vi "Automated Pressure Control v20.vi"() -> ()   [LabVIEW 2011]
uses:
  <vilib>/LabVIEW Interface for Arduino/Type Defs/Pin Mode.ctl
  <vilib>/LabVIEW Interface for Arduino/Type Defs/Arduino Resource.ctl
  <vilib>/LabVIEW Interface for Arduino/Type Defs/Board Type.ctl
  orders/Firgelli motor/LAC_Software_V2/Firgelli Labview Example/Firgelli_LAC_LabVIEWsourceVer8_2/typeDefs/controlValues.ctl
  <vilib>/vision/Avi1.llb/AviRefnum.ctl
  <vilib>/LabVIEW Interface for Arduino/LabVIEW Interface for Arduino.lvlib
  <vilib>/vision/NI_Vision_Development_Module.lvlib
panel:
  out "Balancing":bool
  out "pArray":dbl[](array[numeric])
  in  "Transducer (psi)":dbl(ring)=1.0 items=["+/- .18 psi"=1.0, "+/- .36 psi"=2.0, "+/- 1.08 psi"=3.0]
  in  "Velocity (%)":dbl(slide)=50.0 min=0.0 max=100.0 step=0.01 scale=0.0..100.0 scale format="%02.2f"
  in  "Digital I/O Pin":u8=4
  in  "VentValveOpen?":bool
  out "selected path":path
  out "Capture Video? 2":bool
  out "VidStarted?":bool
  out "loopTimes":dbl[](array[numeric])
  out "Avi Refnum":T1
  in  "Capture Video?":bool
  out "loop exec time (ms)":u32
  out "frameSize":cluster{"Height":i32, "Width":i32}
  out "ROIYDim":dbl
  out "ROIXDim":dbl
  in  "Clear ROI":bool
  in  "Accept ROI":bool
  out "ROI":T2(plugin-control)
  out "error out":errorcluster caption="error"
  in  "Camera ID":u32
  in  "Stopp":bool
  out "FPS":dbl=6.258409738085552
  out "Width":i32=640
  out "Height":i32=480
  in  "Autogain":bool=TRUE
  in  "Master Gain":i32(slide) min=0 max=100 scale=0.0..100.0
  in  "Hotpixel correction":bool
  in  "Blacklevel compensation":bool
  in  "Edge Filter":i32(ring)=2 items=["High"=1, "Low"=2]
  in  "Edge Filter Enable / Disable":bool
  in  "Exposure time":dbl(slide)=33.21525 min=0.045771428571428574 max=49.06697142857143 step=0.045771428571428574 scale=0.045771428571428574..49.06697142857143 scale format="%#.3g"
  in  "Pixel clock":i32(slide)=20 min=5 max=43 scale=5.0..43.0
  in  "Frame rate":dbl(slide)=30.0 min=7.11187838119018 max=20.361314433379523 step=4.577142857142857e-05 scale=7.11187838119018..20.361314433379523 scale format="%^#_3g"
  in  "Blacklevel Offset":i32(slide) min=0 max=255 scale=0.0..255.0
  out "Bits/Pixel":i32=8
  in  "Syringe (mL)":dbl(ring)=2.0 items=[".5 mL"=2.0, "1 mL"=1.0, "3 mL"=3.0]
  out "LastPosition":dbl
  in  "Meas. Pressure":dbl=0.2
  in  "Accuracy (mm)":dbl(slide)=1.0 min=0.0 max=50.0 step=1e-06 scale=0.0..50.0 scale format="%.2f"
  in  "Position (mm) 2":dbl(slide)=40.0 min=0.0 max=50.0 step=0.1 scale=0.0..50.0 scale format="%.2f"
  in  "Position (mm)":dbl(slide)=35.0 min=0.0 max=50.0 step=0.3 scale=0.0..50.0 scale format="%.2f"
  in  "Balance":bool
  out "Pressure (psi)":dbl(graph) caption="Waveform Chart"
  out "Pressure (psi)":dbl
  out "Actuator Position (mm)":dbl(graph)
  in  "updateRate":i32=100 caption="Update Rate (mSec)"
  out "Control Values":T3
  in  "stop":bool
  out "ArduinoError":errorcluster
  out "ArduinoHandle":T4={"VISA resource"="", "Board Type"=enum."Uno", "Connection Type"=enum."USB / Serial", "Bytes Per Packet (15)"=15}
  in  "Valve I/O Pin":u8=2
  in  "Pin Mode":T6=enum."Output"
  in  "VISA resource":refnum<visa-resource-name>="COM6"
  in  "Zero":bool
  out "PressureOffset":dbl
  in  "ValveOpen?":bool
  out "FirgelliError":errorcluster
  out "READ_HANDLE":u32 format="%04x"
  out "WRITE_HANDLE":u32 format="%04x"
  out "DLLver":string caption="DLL Version"
  in  "StartMeasure":bool
  in  "Balance Pressure":dbl=-0.035 min=-1.0 max=0.0 step=0.001
  in  "Initialize":bool
  in  "length":dbl=50.0 caption="Actuator Length (mm)"
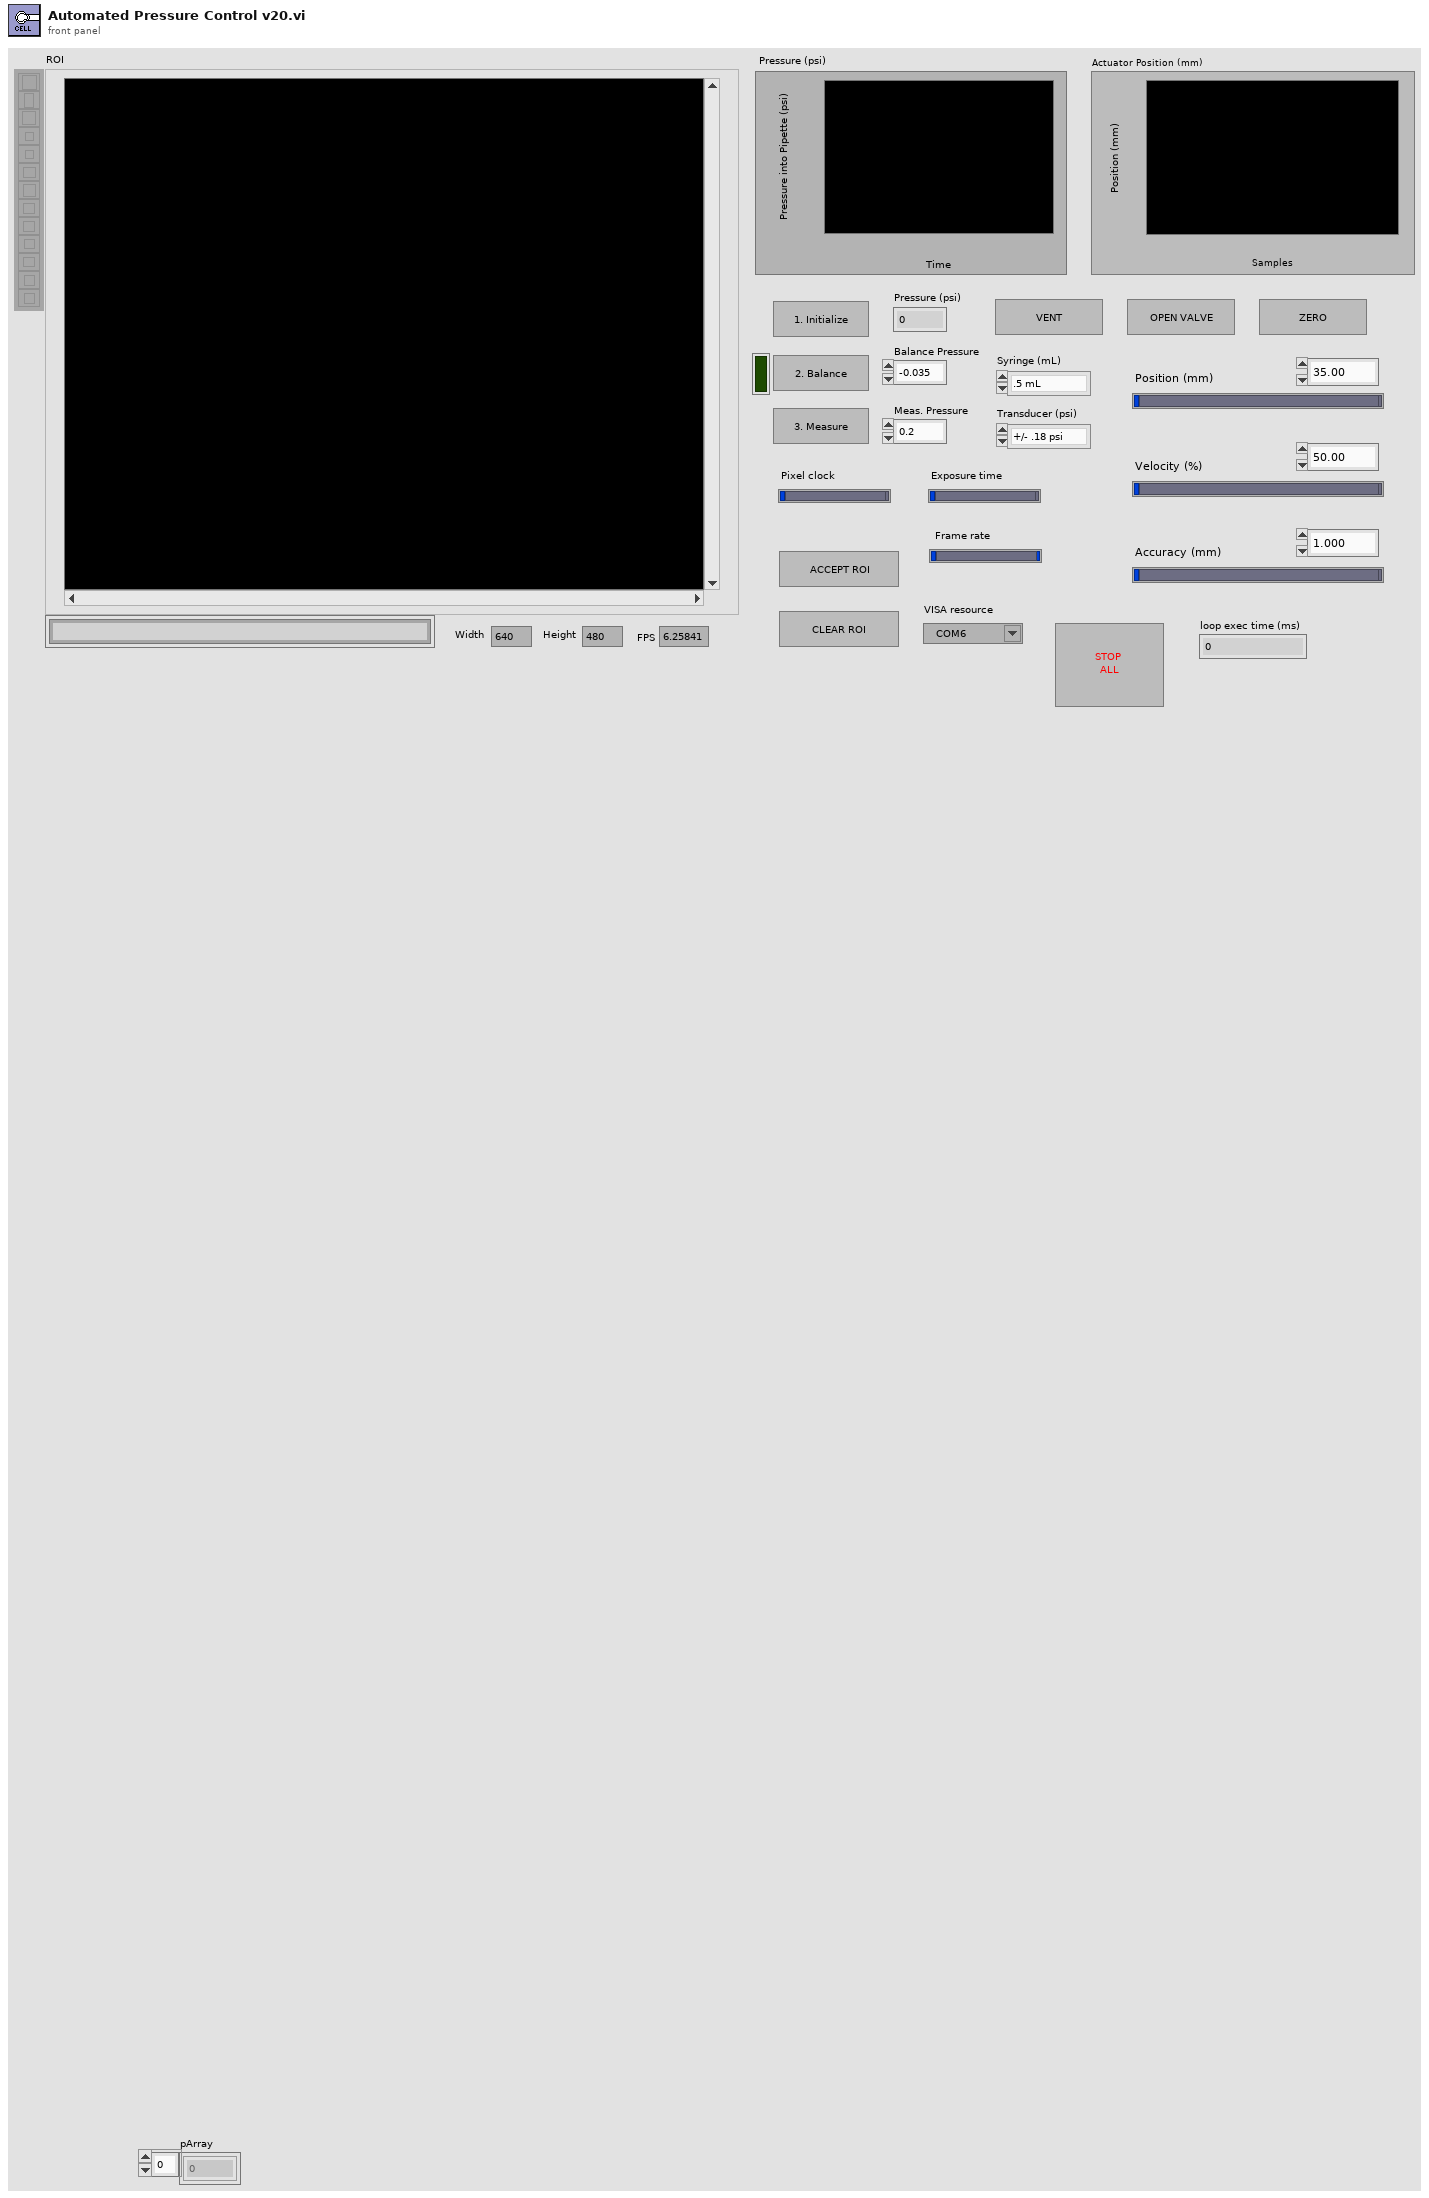
[diagram p1: front panel]
types:
  T1 = typedef "AviRefnum.ctl" = refnum<k1>
  T2 = typedef "IMAQ Image.ctl" = refnum<image>
  T3 = typedef "controlValues.ctl" = cluster{"Position":u16, "Velocity":u16, "Accuracy":u16, "Retract Limit":u16, "Extend Limit":u16}
  T4 = typedef "LabVIEW Interface for Arduino.lvlib/Arduino Resource.ctl" = cluster{"VISA resource":refnum<visa-resource-name>, "Board Type":T5, "Connection Type":enum8{"USB / Serial"}, "Bytes Per Packet (15)":u8}
  T5 = typedef "LabVIEW Interface for Arduino.lvlib/Board Type.ctl" = enum16{"Uno", "Dimuelanove w/Atmega 328", "Mega 2560"}
  T6 = typedef "LabVIEW Interface for Arduino.lvlib/Pin Mode.ctl" = enum8{"Input", "Output"}
  T7 = cluster{"Global Rectangle":i32[], "Contours":cluster{"Contour Type":u32, "ROI Type":u32, "Points":i32[]}[]}
  T8 = cluster{"x1Left":i32, "y1Top":i32, "x2Right":i32, "y2Bottom":i32}
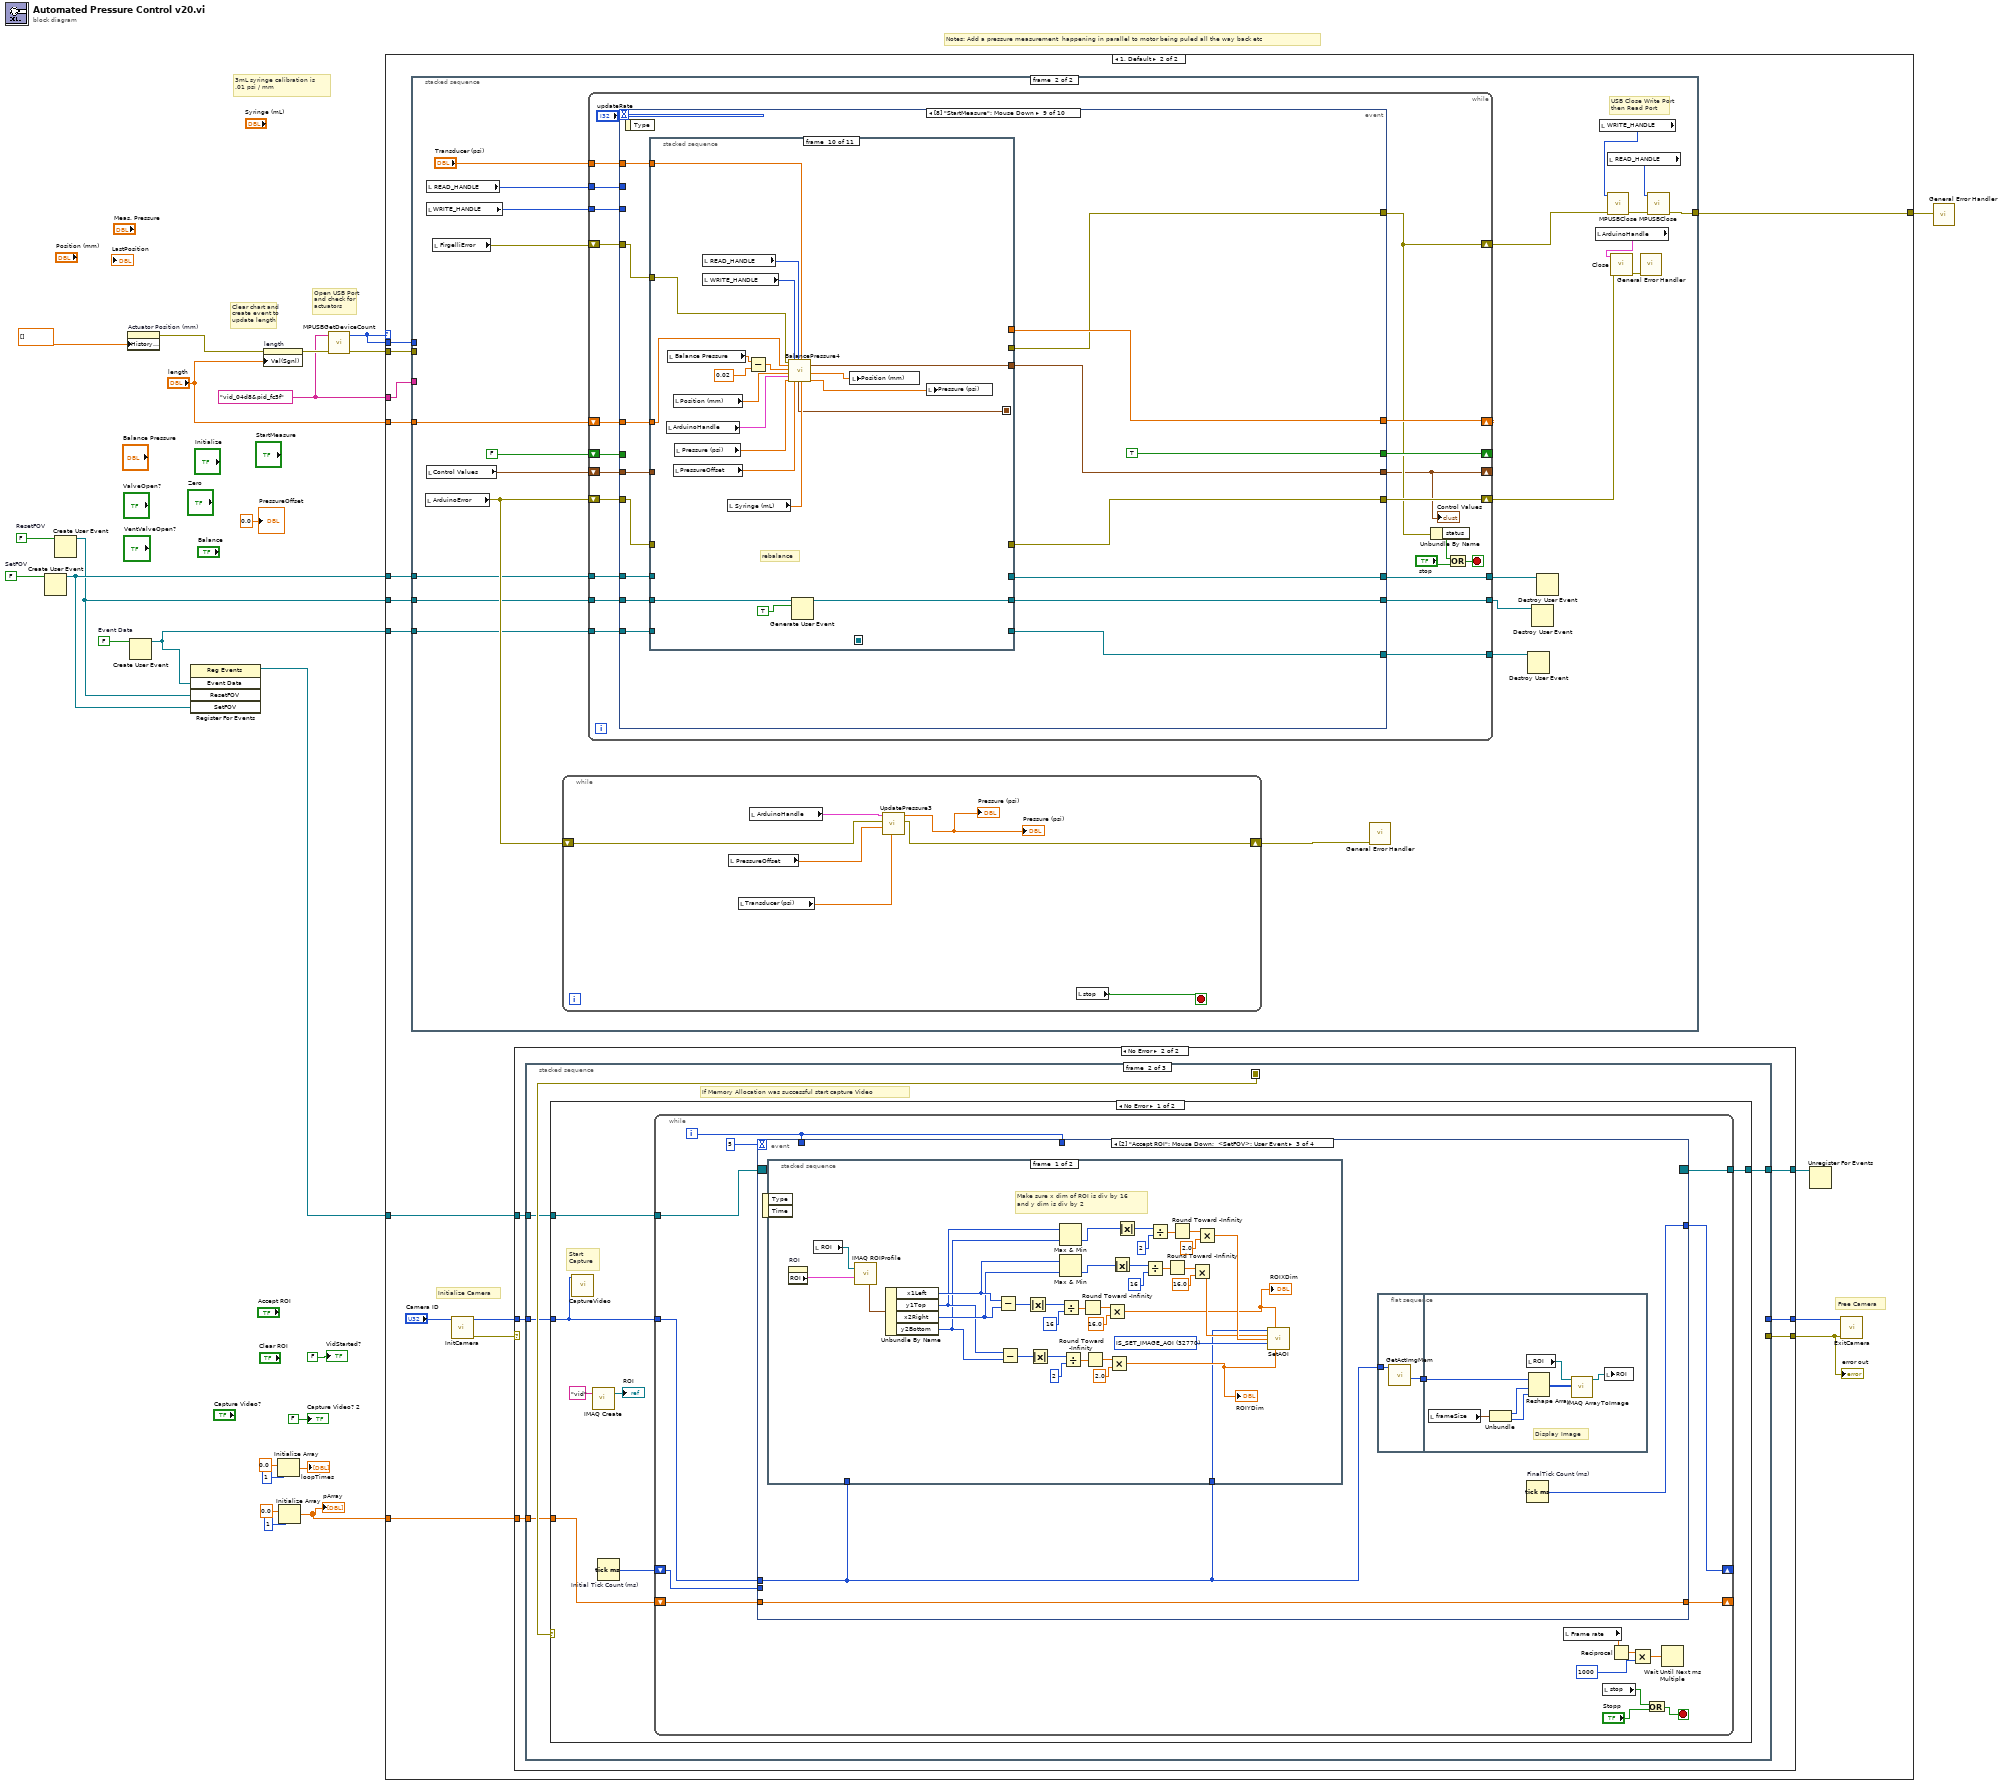
[diagram p0: block diagram]
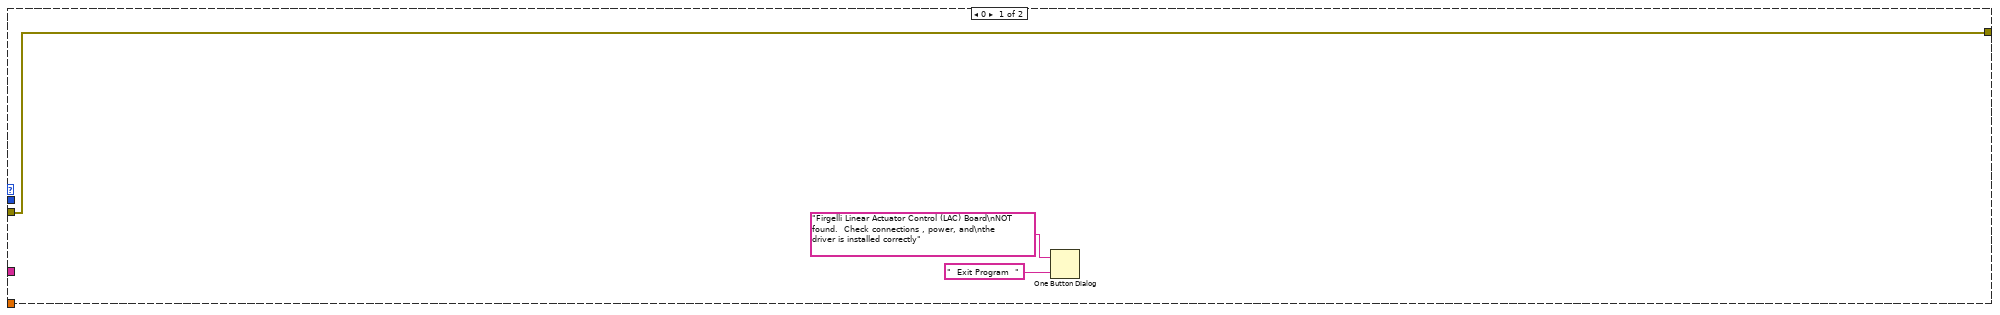
[diagram p2: hidden frame]
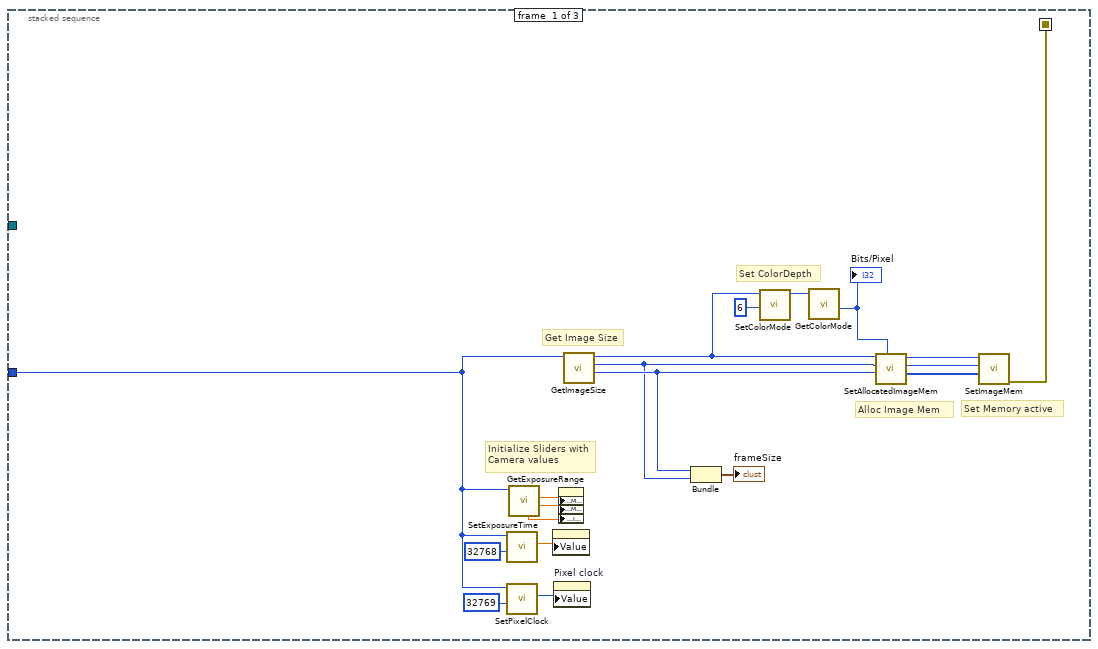
[diagram p4: hidden frame]
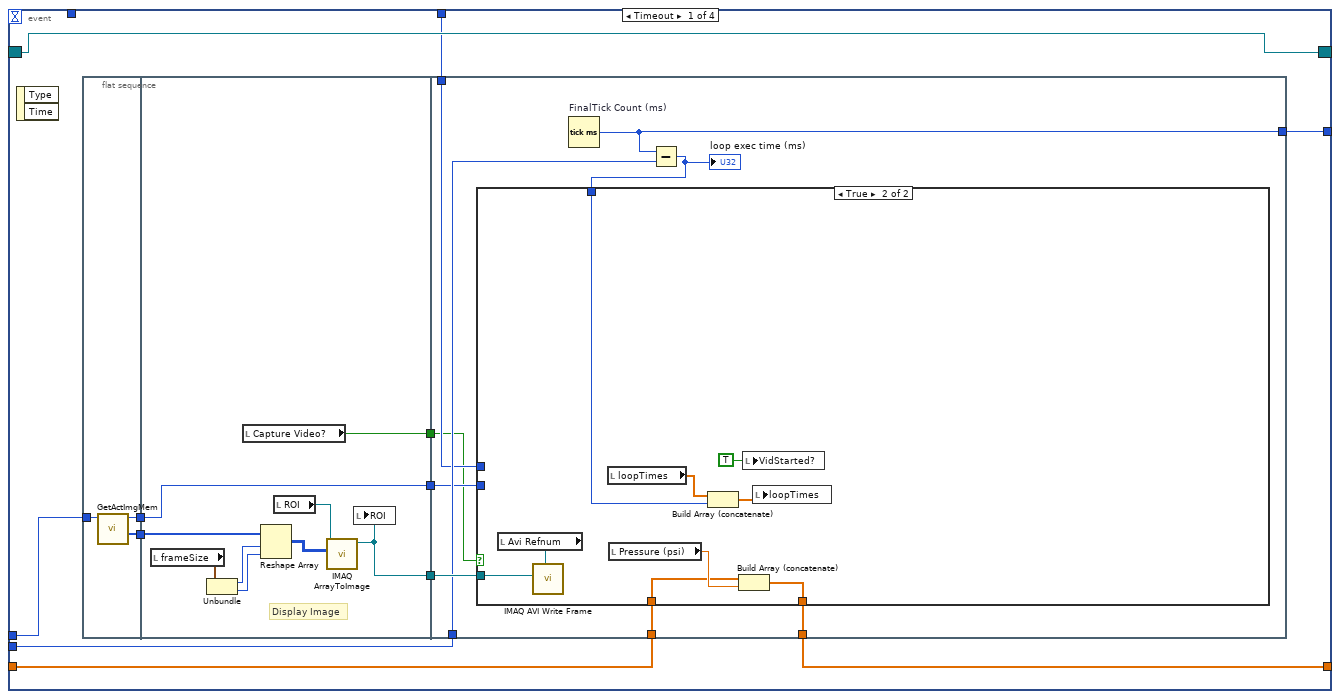
[diagram p5: hidden frame]
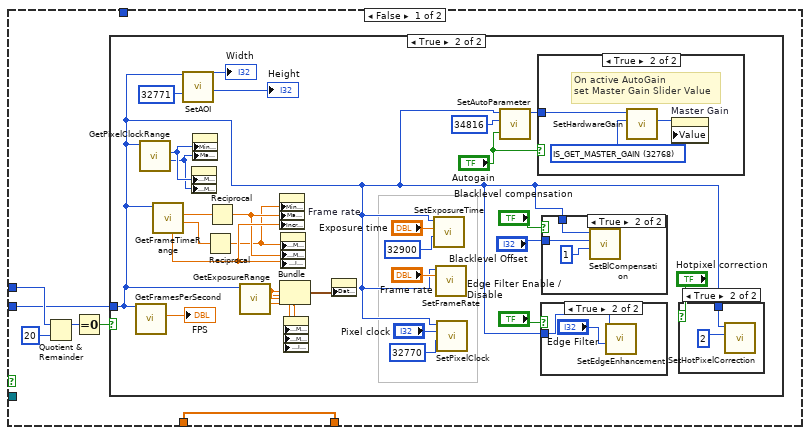
[diagram p6: hidden frame]
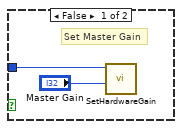
[diagram p8: hidden frame]
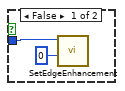
[diagram p9: hidden frame]
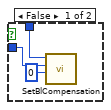
[diagram p10: hidden frame]
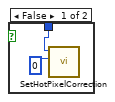
[diagram p11: hidden frame]
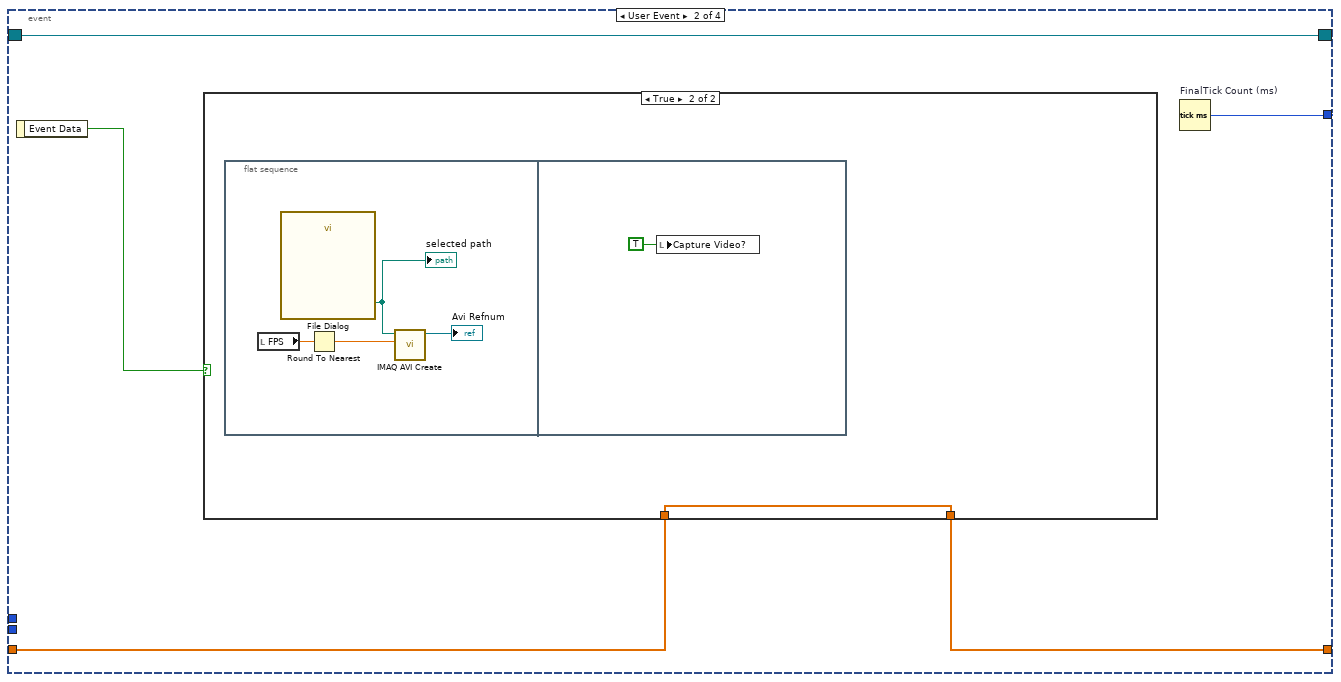
[diagram p12: hidden frame]
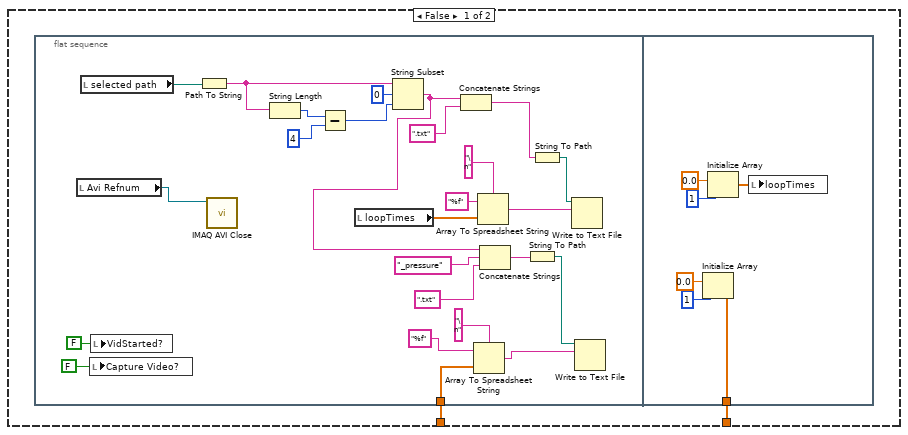
[diagram p13: hidden frame]
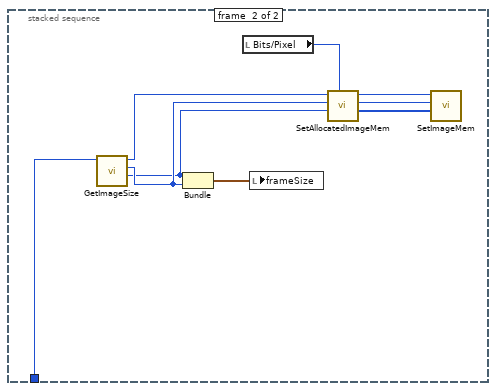
[diagram p14: hidden frame]
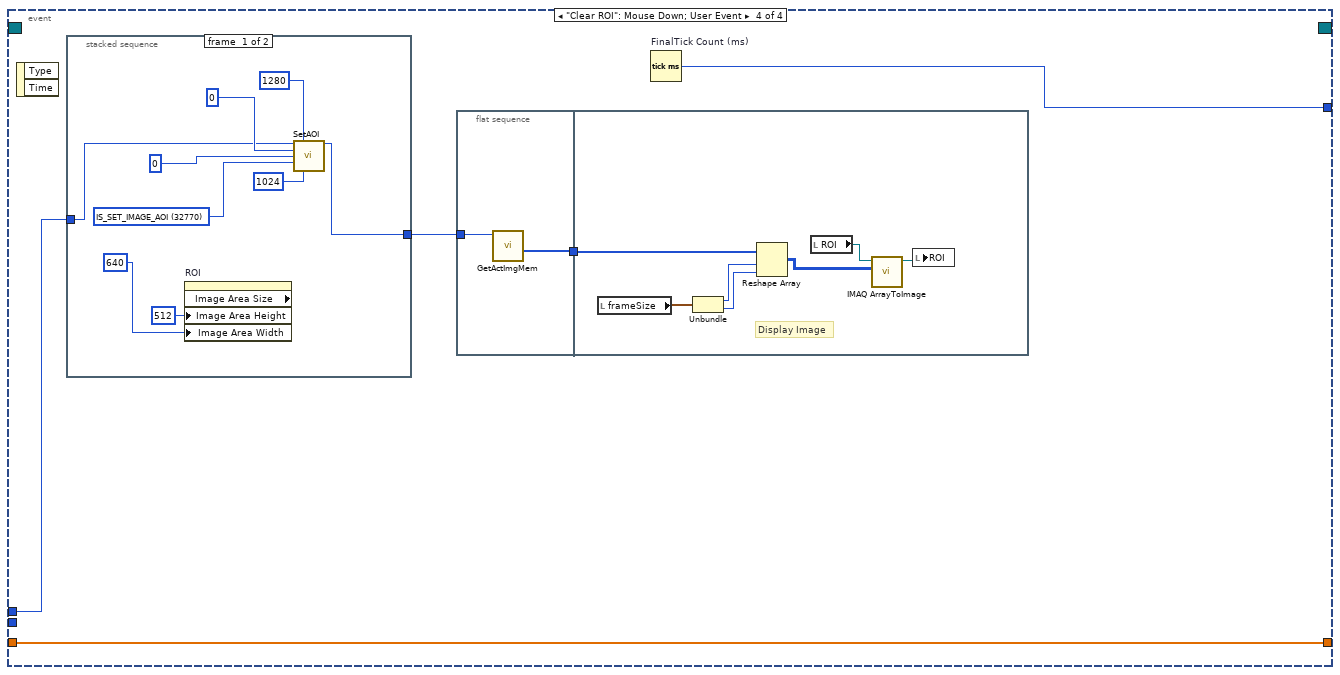
[diagram p15: hidden frame]
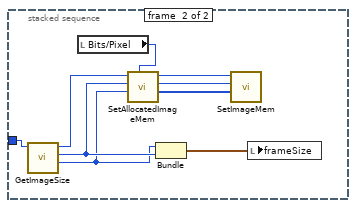
[diagram p16: hidden frame]
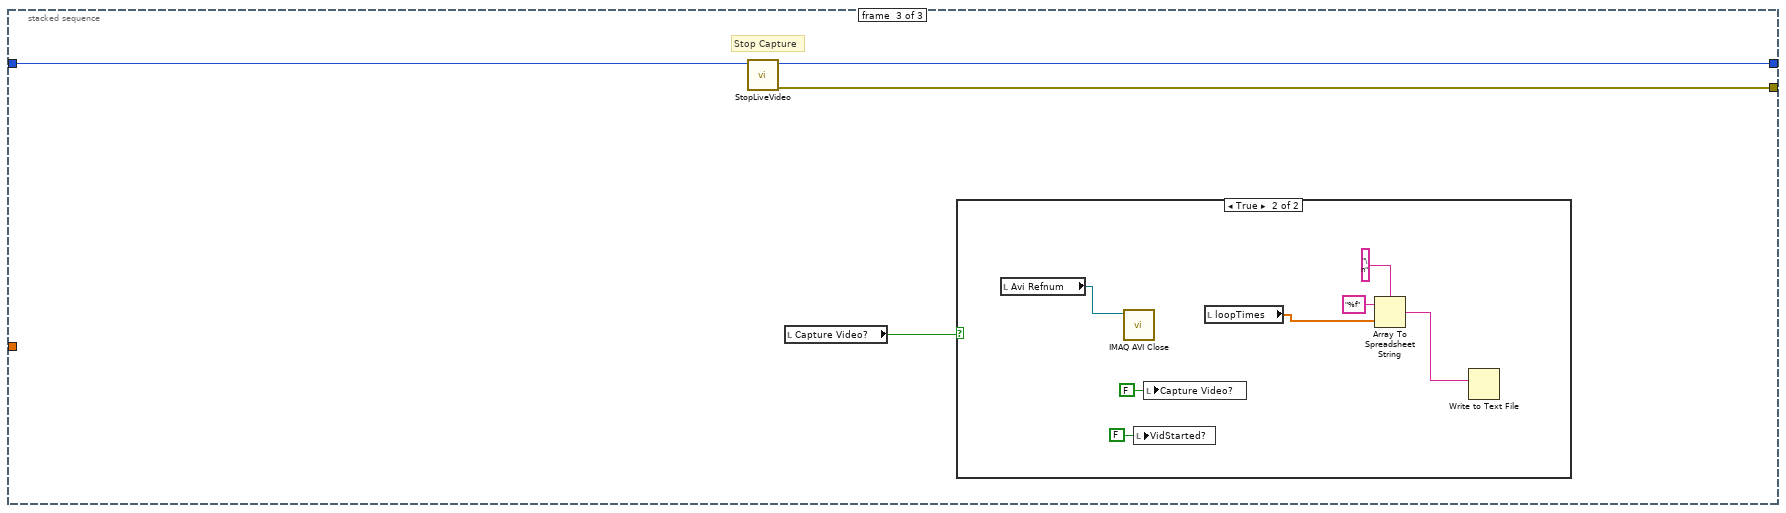
[diagram p18: hidden frame]
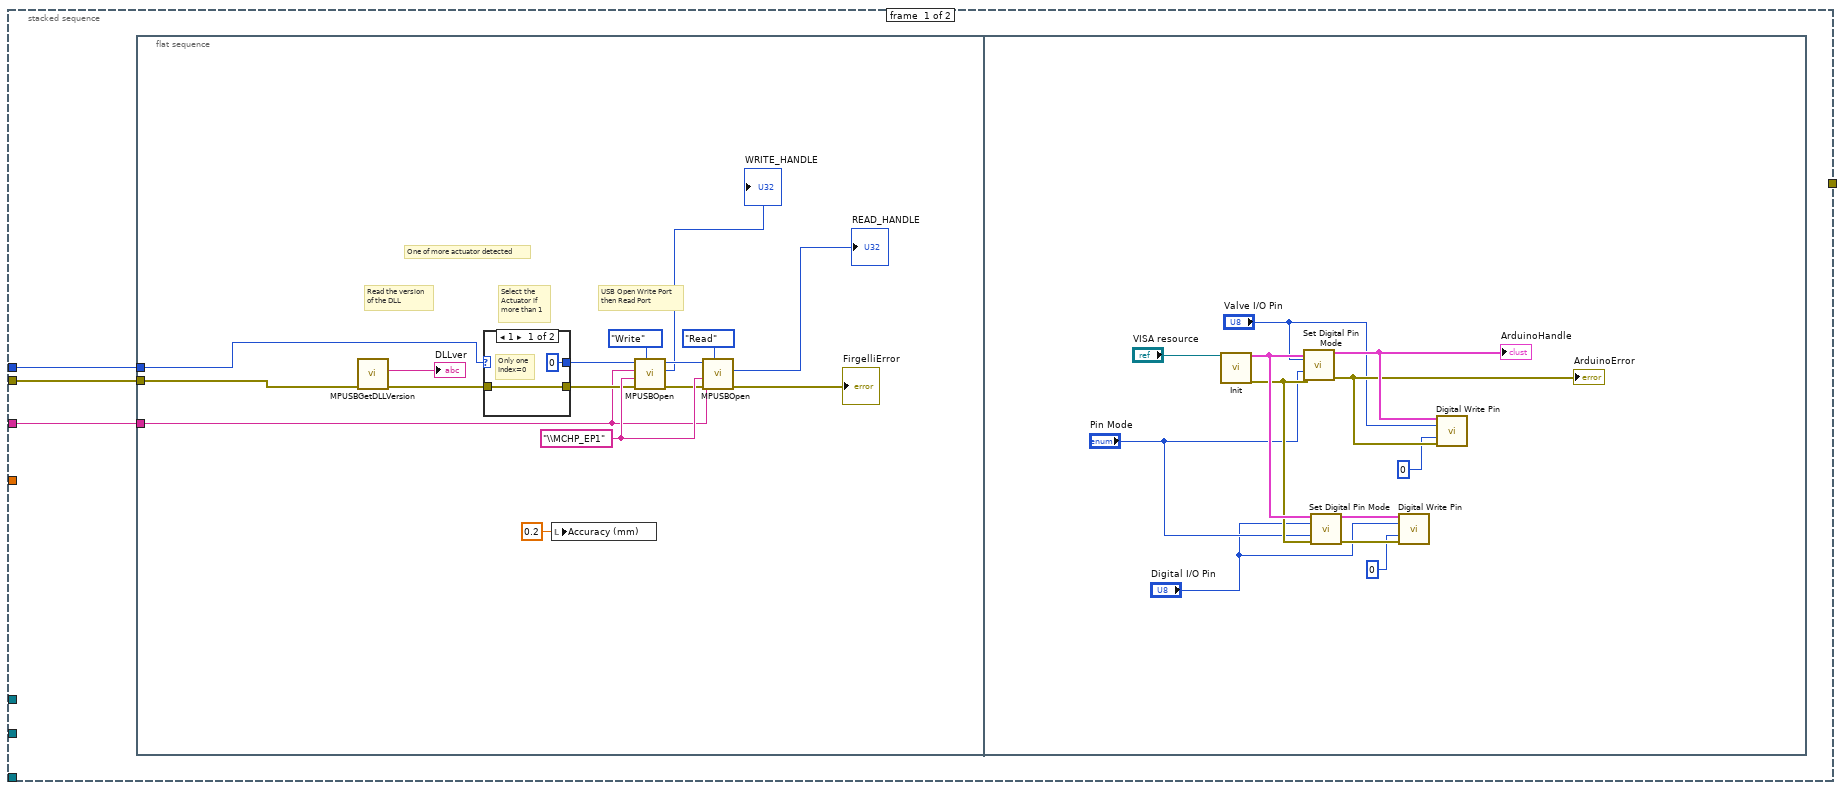
[diagram p20: hidden frame]
diagram:
  w6 = FALSE  # ResetFOV
  w7 = FALSE  # SetFOV
  w10 = FALSE  # Event Data
  w21 = "vid_04d8&pid_fc5f"
  # "3mL syringe calibration is\n.01 psi / mm"
  # "Notes: Add a pressure measurement  happening in parallel to motor being puled all the way back etc"
  # "Open USB Port\nand check for\nactuators"
  # "Clear chart and\ncreate event to \nupdate length"
  n1 = Create User Event(user event datatype=w7) -> (user event=w5:refnum<user-event>)  [unwired: 1 in, 1 out]
  n2 = Create User Event(user event datatype=w6) -> (user event=w4:refnum<user-event>)  [unwired: 1 in, 1 out]
  n3 = property on="Actuator Position (mm)" class="WFChart (strict)"("History Data"=dbl[] []) -> (error out=w22:errorcluster)  [unwired: 2 in, 1 out]
  n4 = Create User Event(user event datatype=w10) -> (user event=w8:refnum<user-event>)  [unwired: 1 in, 1 out]
  n5 = register-events(w8, w4, w5) -> (reference out=w9:refnum<event-registration>)  [unwired: 2 in, 1 out]
  n6 = property on="length" class="DigNum (strict)"(error in=w22, "Val(Sgnl)"="length") -> (error out=w24:errorcluster)  [unwired: 1 in, 1 out]
  n7 = Initialize Array(0.0 ("element"), 1 ("dimension size")) -> (→"loopTimes":dbl[])
  n8 = Initialize Array(0.0 ("element"), 1 ("dimension size")) -> (w1:dbl[])
  "pArray" <- w1
  n9 = call "MPUSBGetDeviceCount.vi"("error in (no error)"=w24, "pVID_PID"=w21) -> ("error out"=w20:errorcluster, "return_value"=w19:u32)  [unwired: 8 out]
  n10 = case shown="1, Default" w19 {
    tunnel: w21 -> [_ w42]
    tunnel: w20 -> [w27 w43]
    tunnel: w19 -> [_ w41]
    tunnel: [w27 w40] -> w18
    tunnel: "length" -> [_ w39]
    tunnel: w9 -> [_ w33]
    tunnel: w8 -> [_ w31]
    tunnel: w5 -> [_ w30]
    tunnel: w4 -> [_ w29]
    tunnel: w1 -> [_ w28]
    frame 0 {
      n11 = One Button Dialog(message="Firgelli Linear Actuator Control (LAC) Board\nNOT found.  Check connections , power, and\nthe driver is installed correctly", button name ("OK")="  Exit Program  ") -> ()  [unwired: 1 out]
    }
    frame 1, Default {
      # "Free Camera"
      # "Initialize Camera"
      n12 = stacked-sequence {
        tunnel: w43 -> [w344 _]
        tunnel: w42 -> [w343 _]
        tunnel: w41 -> [w342 _]
        tunnel: [_ w399] -> w40
        tunnel: w39 -> [_ w391]
        tunnel: w31 -> [_ w388]
        tunnel: w30 -> [_ w383]
        tunnel: w29 -> [_ w382]
        frame #0 {
          n13 = flat-sequence {
            tunnel: w344 -> [w350]
            tunnel: w343 -> [w349]
            tunnel: w342 -> [w348]
            frame #0 {
              w360 = "\\MCHP_EP1" ("pEP")
              # "One of more actuator detected"
              # "Select the\nActuator if\nmore than 1"
              # "Read the version\nof the DLL"
              # "USB Open Write Port\nthen Read Port"
              n14 = call "MPUSBGetDLLVersion.vi"("error in (no error)"=w350) -> ("error out"=w355:errorcluster, "DLLver"=→"DLLver":string)  [unwired: 9 out]
              n15 = case shown="1" w348 {
                selector: w348 -> [_ w363]
                tunnel: w355 -> [w362 w366]
                tunnel: [w362 w365] -> w354
                tunnel: [u32 0 ("Selected") w364] -> w353
                frame 1 {
                  # "Only one\nIndex=0"
                }
                frame Default {
                  n16 = call "actuatorSelect.vi"("error in (no error)"=w366, "Devices"=w363) -> ("error out"=w365:errorcluster, "Selected"=w364:u32)  [unwired: 8 out]
                }
              }
              n17 = local write "Accuracy (mm)"(0.2 ("Accuracy (mm)")) -> ()
              n18 = call "MPUSBOpen.vi"("dwDir"=enum16{"Write", "Read"}."Write", "error in (no error)"=w354, "pEP"=w360, "pVID_PID"=w349, "instance"=w353) -> ("error out"=w357:errorcluster, "HANDLE"=→"WRITE_HANDLE":u32, "instanceOut"=w352:u32)  [unwired: 4 in]
              n19 = call "MPUSBOpen.vi"("dwDir"=enum16{"Write", "Read"}."Read", "error in (no error)"=w357, "pEP"=w360, "pVID_PID"=w349, "instance"=w352) -> ("error out"=→"FirgelliError":errorcluster, "HANDLE"=→"READ_HANDLE":u32)  [unwired: 3 in, 2 out]
            }
            frame #1 {
              n20 = call <vilib>:"Init.vi"("VISA resource"="VISA resource") -> ("Arduino Resource"=w377:T4, "error out"=w376:errorcluster)  [unwired: 17 in]
              n21 = call <vilib>:"Set Digital Pin Mode.vi"("Arduino Resource"=w377, "Digital I/O Pin"="Valve I/O Pin", "Pin Mode (Input)"="Pin Mode", "error in"=w376) -> ("Arduino Resource"=w374:T4, "error out"=w373:errorcluster)  [unwired: 10 in]
              "ArduinoHandle" <- w374
              "ArduinoError" <- w373
              n22 = call <vilib>:"Set Digital Pin Mode.vi"("Arduino Resource"=w377, "Digital I/O Pin"="Digital I/O Pin", "Pin Mode (Input)"="Pin Mode", "error in"=w376) -> ("Arduino Resource"=w371:T4, "error out"=w370:errorcluster)  [unwired: 10 in]
              n23 = call <vilib>:"Digital Write Pin.vi"("Arduino Resource"=w371, "Digital I/O Pin (0)"="Digital I/O Pin", "Value (0)"=u8 0, "error in"=w370) -> ()  [unwired: 10 in, 2 out]
              n24 = call <vilib>:"Digital Write Pin.vi"("Arduino Resource"=w374, "Digital I/O Pin (0)"="Valve I/O Pin", "Value (0)"=u8 0, "error in"=w373) -> ()  [unwired: 10 in, 2 out]
            }
          }
        }
        frame #1 {
          # "USB Close Write Port\nthen Read Port"
          n25 = local read "ArduinoError"() -> (w390:errorcluster)
          n26 = local read "WRITE_HANDLE"() -> (w386:u32)
          n27 = local read "Control Values"() -> (w392:T3)
          n28 = local read "READ_HANDLE"() -> (w387:u32)
          n29 = local read "FirgelliError"() -> (w398:errorcluster)
          n30 = while {
            shift-right: [w406] -> w389
            shift-left: w390 -> [w407]
            stop <- w408 stop-if-true
            n31 = local read "PressureOffset"() -> (w404:dbl)
            n32 = local read "Transducer (psi)"() -> (w402:dbl)
            n33 = local read "ArduinoHandle"() -> (w405:T4)
            n34 = call "UpdatePressure3.vi"("Transducer (psi)"=w402, "PressureOffset"=w404, "Arduino error in"=w407, "ArduinoHandle"=w405) -> ("Arduino error out"=w406:errorcluster, "Pressure (psi)"=→"Pressure (psi)" →"Pressure (psi)":dbl)  [unwired: 6 in]
            n35 = local read "stop"() -> (w408:bool)
          }
          n36 = while {
            shift-right: [w421] -> w384
            shift-left: w398 -> [w428]
            shift-right: [w424] -> w394
            shift-left: w390 -> [w425]
            shift-right: [w422] -> _
            shift-left: FALSE -> [w427]
            shift-right: [w418] -> _
            shift-left: w392 -> [w420]
            shift-right: [w423] -> _
            shift-left: w391 -> [w426]
            tunnel: w388 -> [w417]
            tunnel: [w416] -> w379
            tunnel: w387 -> [w415]
            tunnel: w386 -> [w414]
            tunnel: "Transducer (psi)" -> [w413]
            tunnel: w383 -> [w412]
            tunnel: w382 -> [w411]
            tunnel: [w410] -> w381
            tunnel: [w409] -> w380
            stop <- w429 stop-if-true
            n37 = event shown="[8] \"StartMeasure\": Mouse Down" {
              selector: _ -> [_ _ _ _ _ _ _ _ _ _]
              dyn-events: _ -> [_ _ _ _ _ _ _ _ _ _]
              timeout: "updateRate" -> [_ _ _ _ _ _ _ _ _ _]
              tunnel: w428 -> [w444 w455 w470 w483 w498 w545 w568 w588 w603 w681]
              tunnel: [w442 w445 w469 w481 w490 w545 w568 w588 w601 w680] -> w421
              tunnel: w427 -> [w439 _ _ _ w493 _ w564 w586 _ w678]
              tunnel: w426 -> [w440 w450 w462 w477 w495 w549 w565 w587 w605 w679]
              tunnel: w425 -> [w438 w448 w461 w475 w488 w546 w567 w584 w606 w675]
              tunnel: [w438 w448 w461 w475 w487 w546 w566 w584 w600 w675] -> w424
              tunnel: [w440 w450 w462 w477 w491 w549 w565 w587 w602 w679] -> w423
              tunnel: [w439 TRUE TRUE TRUE w496 TRUE w564 w586 TRUE w678] -> w422
              tunnel: w420 -> [w436 w452 w465 w479 w497 w547 w563 w585 w604 w677]
              tunnel: [w436 w451 w464 w478 w492 w547 w563 w585 w599 w676] -> w418
              tunnel: w417 -> [w437 _ w457 w474 w489 _ w562 w582 w597 w674]
              tunnel: [w437 _ w457 w474 w489 _ w562 w582 w596 w674] -> w416
              tunnel: w415 -> [w435 w447 _ w472 w486 _ _ _ _ w673]
              tunnel: w414 -> [w434 w446 _ w473 w485 _ _ _ _ w672]
              tunnel: w413 -> [_ _ _ _ _ _ _ _ w595 _]
              tunnel: w412 -> [w433 _ _ _ _ _ _ _ w594 _]
              tunnel: w411 -> [w432 _ _ _ _ _ _ _ w593 _]
              tunnel: [w433 _ _ _ _ _ _ _ w592 _] -> w410
              tunnel: [w432 _ _ _ _ _ _ _ w591 _] -> w409
              event Timeout {
                n38 = event-data() -> ()  [unwired: 1 in, 2 out]
                n39 = call "readPosistionFirgelli.vi"("error in (no error)"=w444, "handleIn"=w434) -> ("error out"=w443:errorcluster)  [unwired: 9 out]
                n40 = call "MPUSBRead.vi"("maxLength"=w440, "error in (no error)"=w443, "handleIn"=w435) -> ("error out"=w442:errorcluster, "setValue"=→"Actuator Position (mm)":dbl)  [unwired: 3 in, 4 out]
              }
              event "Velocity (%)": Value Change {
                n41 = event-data() -> ()  [unwired: 1 in, 5 out]
                n42 = call "writeVelocityFirgelli.vi"("error in (no error)"=w455, "Velocity"="Velocity (%)", "handleIn"=w446) -> ("error out"=w454:errorcluster, "regSetting"=w453:u16)  [unwired: 7 out]
                n43 = Bundle By Name(cluster=w452, "Velocity"=w453) -> (w451:T3)
                n44 = call "MPUSBRead.vi"("error in (no error)"=w454, "handleIn"=w447) -> ("error out"=w445:errorcluster)  [unwired: 4 in, 5 out]
              }
              event "Initialize": Mouse Down {
                n45 = event-data() -> ()  [unwired: 1 in, 7 out]
                n46 = local write "Position (mm)"("Position (mm) 2") -> ()
                n47 = local read "WRITE_HANDLE"() -> (w468:u32)
                n48 = local read "READ_HANDLE"() -> (w467:u32)
                n49 = call "writePositionFirgelli.vi"("error in (no error)"=w470, "lengthMax"=w462, "Position (mm)"="Position (mm) 2", "handleIn"=w468) -> ("error out"=w471:errorcluster, "regSetting"=w466:u16)  [unwired: 6 out]
                n50 = call "MPUSBRead.vi"("error in (no error)"=w471, "handleIn"=w467) -> ("error out"=w469:errorcluster)  [unwired: 4 in, 5 out]
                n51 = Bundle By Name(cluster=w465, "Position"=w466) -> (w464:T3)
                n52 = One Button Dialog(message="Connect tubing after\nmotor has reached\ncorrect position", button name ("OK")="OK") -> ()  [unwired: 1 out]
              }
              event "Position (mm)": Value Change {
                n53 = event-data() -> ()  [unwired: 1 in, 5 out]
                n54 = local read "Position (mm)"() -> (w484:dbl)
                n55 = call "writePositionFirgelli.vi"("error in (no error)"=w483, "lengthMax"=w477, "Position (mm)"=w484, "handleIn"=w473) -> ("error out"=w482:errorcluster, "regSetting"=w480:u16)  [unwired: 6 out]
                n56 = call "MPUSBRead.vi"("error in (no error)"=w482, "handleIn"=w472) -> ("error out"=w481:errorcluster)  [unwired: 4 in, 5 out]
                n57 = Bundle By Name(cluster=w479, "Position"=w480) -> (w478:T3)
              }
              event "Balance": Value Change {
                n58 = event-data() -> ("NewVal"=w494:bool)  [unwired: 1 in, 4 out]
                n59 = stacked-sequence {
                  tunnel: w498 -> [_ w516 _]
                  tunnel: w497 -> [_ w515 _]
                  tunnel: w495 -> [_ w513 _]
                  tunnel: w494 -> [_ w512 _]
                  tunnel: w493 -> [_ w511 _]
                  tunnel: [_ w514 _] -> w496
                  tunnel: [_ w510 _] -> w492
                  tunnel: [_ w509 _] -> w491
                  tunnel: [_ w508 _] -> w490
                  tunnel: [_ w507 _] -> w487
                  tunnel: w488 -> [w500 w506 w541]
                  tunnel: w486 -> [_ w505 _]
                  tunnel: w485 -> [_ w504 _]
                  frame #0 {
                    # "open valve"
                    n60 = local read "ArduinoHandle"() -> (w502:T4)
                    n61 = local read "Valve I/O Pin"() -> (w503:u8)
                    n62 = call <vilib>:"Digital Write Pin.vi"("Arduino Resource"=w502, "Digital I/O Pin (0)"=w503, "Value (0)"=u8 5, "error in"=w500) -> ()  [unwired: 10 in, 2 out]
                    "Balancing" <- TRUE ("Balancing")
                  }
                  frame #1 {
                    n63 = case shown="True" w512 {
                      tunnel: w516 -> [w521 w539]
                      tunnel: w515 -> [w519 w533]
                      tunnel: [w521 w532] -> w508
                      tunnel: [w519 w531] -> w510
                      tunnel: [w518 w530] -> w514
                      tunnel: [w517 w529] -> w507
                      tunnel: w513 -> [w520 w528]
                      tunnel: [w520 w528] -> w509
                      tunnel: w511 -> [w518 _]
                      tunnel: w506 -> [w517 _]
                      tunnel: w505 -> [_ w524]
                      tunnel: w504 -> [_ w523]
                      frame False {
                      }
                      frame True {
                        n64 = local read "Position (mm)"() -> (w536:dbl)
                        n65 = local read "ArduinoHandle"() -> (w535:T4)
                        n66 = local read "Balance Pressure"() -> (w538:dbl)
                        n67 = local read "Pressure (psi)"() -> (w537:dbl)
                        n68 = local read "Syringe (mL)"() -> (w525:dbl)
                        n69 = local read "Transducer (psi)"() -> (w522:dbl)
                        n70 = local read "PressureOffset"() -> (w534:dbl)
                        n71 = call "BalancePressure4.vi"("FirgelliError"=w539, "length"=w528, "DesiredPressure"=w538, "Position (mm)"=w536, "ArduinoHandle"=w535, "CurrentPressure"=w537, "WRITE_HANDLE"=w523, "PressureOffset"=w534, "READ_HANDLE"=w524, "Control Values"=w533, "Transducer (psi)"=w522, "Syringe (mL)"=w525) -> ("FirgelliError Out"=w532:errorcluster, "Control Values Out"=w531:T3, "UpdateChart?"=w530:bool, "Position (mm) Out"=w527:dbl, "ArduinoError Out"=w529:errorcluster, "Pressure (psi)"=w526:dbl)  [unwired: 2 in]
                        n72 = local write "Pressure (psi)"(w526) -> ()
                        n73 = local write "Position (mm)"(w527) -> ()
                      }
                    }
                  }
                  frame #2 {
                    w540 = FALSE ("Balance")
                    # "close valve"
                    n74 = local read "ArduinoHandle"() -> (w543:T4)
                    n75 = local read "Valve I/O Pin"() -> (w542:u8)
                    n76 = local write "Balancing"(w540) -> ()
                    n77 = local write "Balance"(w540) -> ()
                    n78 = call <vilib>:"Digital Write Pin.vi"("Arduino Resource"=w543, "Digital I/O Pin (0)"=w542, "Value (0)"=u8 0, "error in"=w541) -> ()  [unwired: 10 in, 2 out]
                  }
                }
              }
              event "VentValveOpen?": Value Change {
                n79 = event-data() -> ("NewVal"=w553:bool)  [unwired: 1 in, 4 out]
                n80 = local read "ArduinoHandle"() -> (w551:T4)
                n81 = local read "ArduinoError"() -> (w550:errorcluster)
                n82 = local read "Digital I/O Pin"() -> (w552:u8)
                n83 = case shown="True" w553 {
                  tunnel: w551 -> [w556 w560]
                  tunnel: w550 -> [w555 w559]
                  tunnel: w552 -> [w554 w558]
                  frame False {
                    n84 = call <vilib>:"Digital Write Pin.vi"("Arduino Resource"=w556, "Digital I/O Pin (0)"=w554, "Value (0)"=u8 0, "error in"=w555) -> ()  [unwired: 10 in, 2 out]
                  }
                  frame True {
                    n85 = call <vilib>:"Digital Write Pin.vi"("Arduino Resource"=w560, "Digital I/O Pin (0)"=w558, "Value (0)"=u8 5, "error in"=w559) -> ()  [unwired: 10 in, 2 out]
                  }
                }
              }
              event "ValveOpen?": Value Change {
                n86 = event-data() -> ("NewVal"=w569:bool)  [unwired: 1 in, 4 out]
                n87 = case shown="False" w569 {
                  tunnel: w567 -> [w573 w578]
                  tunnel: [w572 w577] -> w566
                  frame False {
                    n88 = local read "Valve I/O Pin"() -> (w570:u8)
                    n89 = property on="ValveOpen?" class="Bool"("BoolText.Text"="OPEN VALVE" ("Caption.Text")) -> ()  [unwired: 2 in, 2 out]
                    n90 = local read "ArduinoHandle"() -> (w571:T4)
                    n91 = call <vilib>:"Digital Write Pin.vi"("Arduino Resource"=w571, "Digital I/O Pin (0)"=w570, "Value (0)"=u8 0, "error in"=w573) -> ("error out"=w572:errorcluster)  [unwired: 10 in, 1 out]
                  }
                  frame True {
                    n92 = local read "Valve I/O Pin"() -> (w580:u8)
                    n93 = local read "ArduinoHandle"() -> (w581:T4)
                    n94 = property on="ValveOpen?" class="Bool"("BoolText.Text"="CLOSE VALVE" ("Caption.Text")) -> ()  [unwired: 2 in, 2 out]
                    n95 = call <vilib>:"Digital Write Pin.vi"("Arduino Resource"=w581, "Digital I/O Pin (0)"=w580, "Value (0)"=u8 5, "error in"=w578) -> ("error out"=w577:errorcluster)  [unwired: 10 in, 1 out]
                  }
                }
              }
              event "Zero": Mouse Down {
                n96 = event-data() -> ()  [unwired: 1 in, 7 out]
                n97 = local read "Pressure (psi)"() -> (w590:dbl)
                n98 = local read "PressureOffset"() -> (w583:dbl)
                n99 = Subtract(x=w583, y=w590) -> (x-y=w589:dbl)
                n100 = local write "PressureOffset"(w589) -> ()
              }
              event "StartMeasure": Mouse Down {
                n101 = event-data() -> ()  [unwired: 1 in, 1 out]
                n102 = stacked-sequence {
                  seq-local: [_ w625 _ _ _ _ _ _ _ _ _] -> [_ _ _ _ _ _ _ _ _ w651 _]
                  seq-local: [_ _ w630 _ _ _ _ _ _ _ _] -> [_ _ _ _ _ _ _ w640 _ _ _]
                  tunnel: w606 -> [w607 w615 _ _ _ w635 _ _ _ _ w667]
                  tunnel: w603 -> [_ w618 _ _ _ _ _ _ w644 w654 _]
                  tunnel: w605 -> [_ w617 _ _ _ _ _ _ w645 w653 _]
                  tunnel: w604 -> [_ w616 _ _ _ _ _ _ _ _ _]
                  tunnel: w597 -> [_ _ w631 _ _ _ _ _ _ _ _]
                  tunnel: [_ _ _ _ _ _ _ _ _ w652 _] -> w599
                  tunnel: [_ _ _ _ _ _ _ _ w644 _ _] -> w601
                  tunnel: [_ _ _ _ _ _ _ _ w645 _ _] -> w602
                  tunnel: [_ w615 _ _ _ _ _ _ _ _ _] -> w600
                  tunnel: [_ _ _ _ _ _ _ w641 _ _ _] -> w596
                  tunnel: w595 -> [_ _ _ _ _ _ _ _ _ w650 _]
                  tunnel: w594 -> [_ w613 _ _ _ _ _ _ _ _ _]
                  tunnel: w593 -> [_ _ _ _ _ _ _ _ _ w648 _]
                  tunnel: [_ w612 _ _ _ _ _ _ _ _ _] -> w592
                  tunnel: [_ _ _ _ _ _ _ _ _ w647 _] -> w591
                  frame #0 {
                    # "make sure valve is closed"
                    n103 = local read "Valve I/O Pin"() -> (w609:u8)
                    n104 = local read "ArduinoHandle"() -> (w610:T4)
                    n105 = call <vilib>:"Digital Write Pin.vi"("Arduino Resource"=w610, "Digital I/O Pin (0)"=w609, "Value (0)"=u8 0, "error in"=w607) -> ()  [unwired: 10 in, 2 out]
                  }
                  frame #1 {
                    # "calibrate how far back to move it"
                    # "move motor back"
                    n106 = local read "WRITE_HANDLE"() -> (w621:u32)
                    n107 = local read "Position (mm)"() -> (w620:dbl)
                    n108 = local read "Meas. Pressure"() -> (w629:dbl)
                    n109 = local read "ArduinoHandle"() -> (w628:T4)
                    n110 = local read "Pressure (psi)"() -> (w627:dbl)
                    n111 = local read "PressureOffset"() -> (w626:dbl)
                    n112 = local read "Transducer (psi)"() -> (w611:dbl)
                    n113 = local read "READ_HANDLE"() -> (w622:u32)
                    n114 = local read "Syringe (mL)"() -> (w619:dbl)
                    n115 = local write "LastPosition"(w620) -> ()
                    n116 = call "BalancePressure4.vi"("FirgelliError"=w618, "length"=w617, "DesiredPressure"=w629, "Position (mm)"=w620, "ArduinoHandle"=w628, "CurrentPressure"=w627, "WRITE_HANDLE"=w621, "PressureOffset"=w626, "READ_HANDLE"=w622, "Control Values"=w616, "Transducer (psi)"=w611, "Syringe (mL)"=w619) -> ("Control Values Out"=w625:T3, "Position (mm) Out"=w623:dbl, "Pressure (psi)"=w624:dbl)  [unwired: 2 in, 3 out]
                    n117 = Generate User Event(user event=w613, event data cluster=TRUE ("ResetFOV")) -> (user event out=w612:refnum<user-event>)  [unwired: 1 in, 1 out]
                    n118 = local write "Position (mm)"(w623) -> ()
                    n119 = local write "Pressure (psi)"(w624) -> ()
                  }
                  frame #2 {
                    n120 = Generate User Event(user event=w631, event data cluster=TRUE ("event data")) -> (user event out=w630:refnum<user-event>)  [unwired: 1 in, 1 out]
                  }
                  frame #3 {
                    # "Once CaptureVideo is T, the \nvideo is started. Once first \nframe is captured, the loop\nends and the next frame starts"
                    # "Start recording\nvideo here"
                    n121 = while {
                      stop <- w633 stop-if-true
                      n122 = local read "VidStarted?"() -> (w633:bool)
                    }
                  }
                  frame #4 {
                    n123 = Wait (ms)(milliseconds to wait=u32 1000) -> ()  [unwired: 1 out]
                  }
                  frame #5 {
                    # "open valve"
                    n124 = local read "Valve I/O Pin"() -> (w637:u8)
                    n125 = local read "ArduinoHandle"() -> (w638:T4)
                    n126 = call <vilib>:"Digital Write Pin.vi"("Arduino Resource"=w638, "Digital I/O Pin (0)"=w637, "Value (0)"=u8 5, "error in"=w635) -> ()  [unwired: 10 in, 2 out]
                  }
                  frame #6 {
                    n127 = Wait (ms)(milliseconds to wait=u32 5000) -> ()  [unwired: 1 out]
                  }
                  frame #7 {
                    n128 = Wait (ms)(milliseconds to wait=u32 2000) -> ()  [unwired: 1 out]
                    n129 = Generate User Event(user event=w640, event data cluster=FALSE ("Capture Video?")) -> (user event out=w641:refnum<user-event>)  [unwired: 1 in, 1 out]
                  }
                  frame #8 {
                    # "stop video"
                    n130 = while {
                      stop <- w646 continue-if-true
                      n131 = local read "VidStarted?"() -> (w646:bool)
                    }
                  }
                  frame #9 {
                    # "rebalance"
                    n132 = local read "ArduinoHandle"() -> (w665:T4)
                    n133 = local read "Balance Pressure"() -> (w657:dbl)
                    n134 = local read "Position (mm)"() -> (w666:dbl)
                    n135 = local read "PressureOffset"() -> (w663:dbl)
                    n136 = local read "Pressure (psi)"() -> (w664:dbl)
                    n137 = local read "READ_HANDLE"() -> (w659:u32)
                    n138 = local read "WRITE_HANDLE"() -> (w660:u32)
                    n139 = local read "Syringe (mL)"() -> (w658:dbl)
                    n140 = Subtract(x=w657, y=0.02) -> (x-y=w655:dbl)
                    n141 = call "BalancePressure4.vi"("FirgelliError"=w654, "length"=w653, "DesiredPressure"=w655, "Position (mm)"=w666, "ArduinoHandle"=w665, "CurrentPressure"=w664, "WRITE_HANDLE"=w660, "PressureOffset"=w663, "READ_HANDLE"=w659, "Control Values"=w651, "Transducer (psi)"=w650, "Syringe (mL)"=w658) -> ("Control Values Out"=w652:T3, "Position (mm) Out"=w662:dbl, "Pressure (psi)"=w661:dbl)  [unwired: 2 in, 3 out]
                    n142 = Generate User Event(user event=w648, event data cluster=TRUE ("ResetFOV")) -> (user event out=w647:refnum<user-event>)  [unwired: 1 in, 1 out]
                    n143 = local write "Position (mm)"(w662) -> ()
                    n144 = local write "Pressure (psi)"(w661) -> ()
                  }
                  frame #10 {
                    # "close valve"
                    n145 = local read "ArduinoHandle"() -> (w669:T4)
                    n146 = local read "Valve I/O Pin"() -> (w668:u8)
                    n147 = call <vilib>:"Digital Write Pin.vi"("Arduino Resource"=w669, "Digital I/O Pin (0)"=w668, "Value (0)"=u8 0, "error in"=w667) -> ()  [unwired: 10 in, 2 out]
                  }
                }
              }
              event "Accuracy (mm)": Value Change {
                n148 = event-data() -> ()  [unwired: 1 in, 5 out]
                n149 = call "writeAccuracyFirgelli.vi"("error in (no error)"=w681, "maxLength"=w679, "accuracy"="Accuracy (mm)", "handleIn"=w672) -> ("error out"=w682:errorcluster, "regSetting"=w683:u16)  [unwired: 6 out]
                n150 = Bundle By Name(cluster=w677, "Accuracy"=w683) -> (w676:T3)
                n151 = call "MPUSBRead.vi"("error in (no error)"=w682, "handleIn"=w673) -> ("error out"=w680:errorcluster)  [unwired: 4 in, 5 out]
              }
            }
            "Control Values" <- w418
            n152 = Unbundle By Name(w421) -> ("status"=w430:bool)
            n153 = Or(x=w430, y="stop") -> (x .or. y?=w429:bool)
          }
          n154 = call <vilib>:"General Error Handler.vi"("error in (no error)"=w389) -> ()  [unwired: 1 in, 14 out]
          n155 = Destroy User Event(user event=w379) -> ()  [unwired: 1 in, 1 out]
          n156 = Destroy User Event(user event=w380) -> ()  [unwired: 1 in, 1 out]
          n157 = Destroy User Event(user event=w381) -> ()  [unwired: 1 in, 1 out]
          n158 = local read "ArduinoHandle"() -> (w395:T4)
          n159 = local read "WRITE_HANDLE"() -> (w397:u32)
          n160 = call "MPUSBClose.vi"("error in (no error)"=w384, "handle"=w397) -> ("error out"=w401:errorcluster)  [unwired: 1 in, 8 out]
          n161 = local read "READ_HANDLE"() -> (w396:u32)
          n162 = call <vilib>:"Close.vi"("Arduino Resource"=w395, "error in"=w394) -> ("error out"=w400:errorcluster)  [unwired: 13 in]
          n163 = call <vilib>:"General Error Handler.vi"("error in (no error)"=w400) -> ()  [unwired: 1 in, 14 out]
          n164 = call "MPUSBClose.vi"("error in (no error)"=w401, "handle"=w396) -> ("error out"=w399:errorcluster)  [unwired: 1 in, 8 out]
        }
      }
      n165 = call "InitCamera.vi"("Camera ID"="Camera ID") -> ("error out"=w35:errorcluster, "Camera Handle Out"=w36:u32)  [unwired: 9 in]
      n166 = case shown="No Error" w35 {
        selector: w35 -> [w45 _]
        tunnel: [w46 w52] -> w38
        tunnel: w36 -> [w46 w51]
        tunnel: [w45 w50] -> w34
        tunnel: w33 -> [w44 w49]
        tunnel: [w44 w48] -> w32
        tunnel: w28 -> [_ w47]
        frame Error {
        }
        frame No Error {
          n167 = stacked-sequence {
            seq-local: [w68 _ _] -> [_ w76 _]
            tunnel: w51 -> [w59 w75 w334]
            tunnel: [_ _ w333] -> w52
            tunnel: [_ _ w332] -> w50
            tunnel: w49 -> [_ w74 _]
            tunnel: [_ w73 _] -> w48
            tunnel: w47 -> [_ w72 _]
            frame #0 {
              # "Set Memory active"
              # "Alloc Image Mem"
              # "Set ColorDepth"
              # "Initialize Sliders with\nCamera values"
              # "Get Image Size"
              n168 = call "SetExposureTime.vi"("Mode"=u16 32768, "Camera Handle In"=w59) -> ("new exposure time"=w63:dbl)  [unwired: 7 in, 2 out]
              n169 = call "SetPixelClock.vi"("Mode"=32769, "Camera Handle In"=w59) -> ("Value"=w62:i32)  [unwired: 7 in, 2 out]
              n170 = call "GetExposureRange.vi"("Camera Handle In"=w59) -> ("max"=w65:dbl, "min"=w66:dbl, "intervall"=w64:dbl)  [unwired: 6 in, 2 out]
              n171 = property on="Exposure time" class="Slide (strict)"("Value"=w63) -> ()  [unwired: 2 in, 2 out]
              n172 = property on="Pixel clock" class="Slide (strict)"("Value"=w62) -> ()  [unwired: 2 in, 2 out]
              n173 = property on="Exposure time" class="Schieberegler (strikt)"("Scale.Minimum"=w66, "Scale.Maximum"=w65, "Scale.Increment"=w64) -> ()  [unwired: 2 in, 2 out]
              n174 = call "GetImageSize.vi"("Camera Handle In"=w59) -> ("Height"=w55:i32, "Width"=w54:i32, "Camera Handle Out"=w67:u32)  [unwired: 8 in]
              n175 = Bundle("Height"=w55, "Width"=w54) -> (→"frameSize":cluster{"Height":i32, "Width":i32})  [unwired: 1 in]
              n176 = call "SetColorMode.vi"("Mode"=6, "Camera Handle In"=w67) -> ("Camera Handle Out"=w58:u32)  [unwired: 8 in, 1 out]
              n177 = call "GetColorMode.vi"("Camera Handle In"=w58) -> ("Bits/Pixel"=w56:i32)  [unwired: 8 in, 2 out]
              "Bits/Pixel" <- w56
              n178 = call "SetAllocatedImageMem.vi"("BitsPixel"=w56, "Height"=w55, "Width"=w54, "Camera Handle In"=w67) -> ("Image Memory Out"=w69:u8[], "Memory ID Out"=w70:i32, "Camera Handle Out"=w71:u32)  [unwired: 3 in, 2 out]
              n179 = call "SetImageMem.vi"("Image Memory In"=w69, "Memory ID In"=w70, "Camera Handle In"=w71) -> ("error out"=w68:errorcluster)  [unwired: 5 in, 3 out]
            }
            frame #1 {
              # "If Memory Allocation was successful start capture Video"
              n180 = case shown="No Error" w76 {
                tunnel: w75 -> [w83 _]
                tunnel: w74 -> [w79 w330]
                tunnel: [w78 w330] -> w73
                tunnel: w72 -> [w77 _]
                frame No Error {
                  # "Start\nCapture"
                  n181 = call "CaptureVideo.vi"("Camera Handle In"=w83) -> ()  [unwired: 9 in, 2 out]
                  n182 = call "IMAQ Create"("Image Name"="vid") -> ("New Image"=→"ROI":T2)  [unwired: 4 in, 1 out]
                  n183 = Tick Count (ms) "Initial Tick Count (ms)"() -> (millisecond timer value=w80:u32)
                  n184 = while {
                    tunnel: w83 -> [w84]
                    shift-right: [w93] -> _
                    shift-left: w80 -> [w94]
                    tunnel: w79 -> [w92]
                    tunnel: [w91] -> w78
                    shift-right: [w86] -> _
                    shift-left: w77 -> [w87]
                    i -> [w85]
                    stop <- w90 stop-if-true
                    n185 = event shown="[2] \"Accept ROI\": Mouse Down;  <SetFOV>: User Event" {
                      selector: w92 -> [w107 w199 _ _]
                      dyn-events: [w107 w199 _ _] -> w91
                      timeout: 5 -> [_ _ _ _]
                      tunnel: w85 -> [_ _ _ _]
                      tunnel: w94 -> [w108 _ _ _]
                      tunnel: [w109 w195 w240 w300] -> w93
                      tunnel: w87 -> [w106 w197 w241 w301]
                      tunnel: [w105 w196 w241 w301] -> w86
                      tunnel: w85 -> [w104 _ _ _]
                      tunnel: w84 -> [w101 _ w239 w299]
                      event Timeout {
                        n186 = event-data() -> ()  [unwired: 1 in, 2 out]
                        n187 = flat-sequence {
                          tunnel: [w114] -> w111
                          tunnel: w101 -> [w113]
                          tunnel: [w112] -> w103
                          tunnel: w111 -> [w120]
                          tunnel: [w117] -> w110
                          tunnel: w103 -> [w116]
                          tunnel: [w116] -> w102
                          tunnel: [w115] -> w100
                          tunnel: w110 -> [w132]
                          tunnel: w108 -> [w131]
                          tunnel: [w125] -> w109
                          tunnel: w106 -> [w129]
                          tunnel: [w128] -> w105
                          tunnel: w104 -> [w127]
                          tunnel: w102 -> [w126]
                          tunnel: w100 -> [w124]
                          frame #0 {
                            n188 = call "GetActImgMem.vi"("Camera Handle In"=w113) -> ("Image Memory Out"=w114:u8[], "Camera Handle Out"=w112:u32)  [unwired: 7 in, 2 out]
                          }
                          frame #1 {
                            # "Display Image"
                            n189 = local read "frameSize"() -> (w118:cluster{"Height":i32, "Width":i32})
                            n190 = Unbundle(w118) -> ("Height"=w123:i32, "Width"=w122:i32)
                            n191 = local read "Capture Video?"() -> (w115:bool)
                            n192 = Reshape Array(w120, w123, w122) -> (w119:u8[][])
                            n193 = local read "ROI"() -> (w121:T2)
                            n194 = call "IMAQ ArrayToImage"("Image Pixels (U8)"=w119, "Image"=w121) -> ("Image Out"=w117:T2)  [unwired: 8 in, 1 out]
                            n195 = local write "ROI"(w117) -> ()
                          }
                          frame #2 {
                            n196 = Tick Count (ms) "FinalTick Count (ms)"() -> (millisecond timer value=w125:u32)
                            n197 = Subtract(x=w125, y=w131) -> (x-y=w130:u32)
                            "loop exec time (ms)" <- w130
                            n198 = case shown="True" w124 {
                              tunnel: w132 -> [_ w193]
                              tunnel: w130 -> [_ w192]
                              tunnel: w129 -> [w138 w187]
                              tunnel: [w138 w186] -> w128
                              tunnel: w127 -> [w135 _]
                              tunnel: w126 -> [w133 _]
                              frame False {
                                n199 = Quotient & Remainder(x=w135, y=20) -> (x-y*floor(x/y)=w137:i32)  [unwired: 1 out]
                                n200 = Equal To 0?(x=w137) -> (x = 0?=w134:bool)
                                n201 = case shown="True" w134 {
                                tunnel: w133 -> [_ w139]
                                frame False {
                                }
                                frame True {
                                n202 = call "GetFramesPerSecond.vi"("Camera Handle In"=w139) -> ("FPS"=→"FPS":dbl)  [unwired: 8 in, 2 out]
                                n203 = call "GetPixelClockRange.vi"("Camera Handle In"=w139) -> ("Max"=w155:i32, "Min"=w156:i32)  [unwired: 7 in, 2 out]
                                n204 = call "GetFrameTimeRange.vi"("Camera Handle In"=w139) -> ("max"=w157:dbl, "min"=w158:dbl, "interval"=w161:dbl)  [unwired: 6 in, 2 out]
                                n205 = call "SetAOI.vi"("Camera Handle In"=w139, "Mode"=32771) -> ("Width Out"=→"Width":i32, "Height Out"=→"Height":i32)  [unwired: 8 in, 4 out]
                                n206 = property on="Pixel clock" class="Schieberegler (strikt)"("Scale.Minimum"=w156, "Scale.Maximum"=w155) -> ()  [unwired: 2 in, 2 out]
                                n207 = property on="Pixel clock" class="Schieberegler (strikt)"("Minimum"=w156, "Maximum"=w155) -> ()  [unwired: 2 in, 2 out]
                                n208 = Reciprocal(x=w157) -> (1/x=w159:dbl)
                                n209 = Reciprocal(x=w158) -> (1/x=w160:dbl)
                                n210 = call "GetExposureRange.vi"("Camera Handle In"=w139) -> ("max"=w164:dbl, "min"=w163:dbl, "intervall"=w165:dbl)  [unwired: 6 in, 2 out]
                                n211 = property on="Frame rate" class="Schieberegler (strikt)"("Minimum"=w159, "Maximum"=w160, "Increment"=w161) -> ()  [unwired: 2 in, 2 out]
                                n212 = Bundle("min"=w163, "max"=w164, "intervall"=w165) -> (w162:cluster{"min":dbl, "max":dbl, "intervall":dbl})  [unwired: 1 in]
                                n213 = property on="Frame rate" class="Schieberegler (strikt)"("Scale.Minimum"=w159, "Scale.Maximum"=w160, "Scale.Increment"=w161) -> ()  [unwired: 2 in, 2 out]
                                n214 = property on="Exposure time" class="Schieberegler (strikt)"("Scale.Minimum"=w163, "Scale.Maximum"=w164, "Scale.Increment"=w165) -> ()  [unwired: 2 in, 2 out]
                                n215 = property on="Exposure time" class="Schieberegler (strikt)"("Data Range"=w162) -> ()  [unwired: 2 in, 2 out]
                                n216 = call "SetExposureTime.vi"("Mode"=u16 32900, "Exposure Time"="Exposure time", "Camera Handle In"=w139) -> ()  [unwired: 6 in, 3 out]
                                n217 = call "SetFrameRate.vi"("FPS"="Frame rate", "Camera Handle In"=w139) -> ()  [unwired: 7 in, 3 out]
                                n218 = call "SetPixelClock.vi"("Mode"=32770, "Pixel Clock"="Pixel clock", "Camera Handle In"=w139) -> ()  [unwired: 6 in, 3 out]
                                n219 = call "SetAutoParameter.vi"("enable"="Autogain", "Param"=34816, "Camera Handle In"=w139) -> ("Camera Handle Out"=w141:u32)  [unwired: 6 in, 2 out]
                                n220 = case shown="True" "Autogain" {
                                tunnel: w141 -> [w167 w170]
                                frame False {
                                # "Set Master Gain"
                                n221 = call "SetHardwareGain.vi"("Master Gain"="Master Gain", "Camera Handle In"=w167) -> ()  [unwired: 7 in, 3 out]
                                }
                                frame True {
                                w169 = 32768 items=["IS_GET_MASTER_GAIN"=32768]
                                # "On active AutoGain\nset Master Gain Slider Value"
                                n222 = call "SetHardwareGain.vi"("Mode"=w169, "Camera Handle In"=w170) -> ("Value"=w171:i32)  [unwired: 7 in, 2 out]
                                n223 = property on="Master Gain" class="Slide (strict)"("Value"=w171) -> ()  [unwired: 2 in, 2 out]
                                }
                                }
                                n224 = case shown="True" "Edge Filter Enable / Disable" {
                                tunnel: w139 -> [w172 w174]
                                frame False {
                                n225 = call "SetEdgeEnhancement.vi"("Mode"=0, "Camera Handle In"=w172) -> ()  [unwired: 8 in, 2 out]
                                }
                                frame True {
                                n226 = call "SetEdgeEnhancement.vi"("Mode"="Edge Filter", "Camera Handle In"=w174) -> ()  [unwired: 8 in, 2 out]
                                }
                                }
                                n227 = case shown="True" "Blacklevel compensation" {
                                tunnel: "Blacklevel Offset" -> [w177 w180]
                                tunnel: w139 -> [w176 w179]
                                frame False {
                                n228 = call "SetBlCompensation.vi"("Mode"=0, "offset"=w177, "Camera Handle In"=w176) -> ()  [unwired: 6 in, 3 out]
                                }
                                frame True {
                                n229 = call "SetBlCompensation.vi"("Mode"=1, "offset"=w180, "Camera Handle In"=w179) -> ()  [unwired: 6 in, 3 out]
                                }
                                }
                                n230 = case shown="True" "Hotpixel correction" {
                                tunnel: w139 -> [w182 w184]
                                frame False {
                                n231 = call "SetHotPixelCorrection.vi"("Mode"=0, "Camera Handle In"=w182) -> ()  [unwired: 7 in, 3 out]
                                }
                                frame True {
                                n232 = call "SetHotPixelCorrection.vi"("Mode"=2, "Camera Handle In"=w184) -> ()  [unwired: 7 in, 3 out]
                                }
                                }
                                }
                                }
                              }
                              frame True {
                                n233 = local read "Avi Refnum"() -> (w194:T1)
                                n234 = call "IMAQ AVI Write Frame"("Image"=w193, "Avi Refnum"=w194) -> ()  [unwired: 8 in, 2 out]
                                n235 = local read "loopTimes"() -> (w191:dbl[])
                                n236 = local read "Pressure (psi)"() -> (w188:dbl)
                                n237 = Build Array (concatenate)(w191, w192) -> (w190:dbl[])
                                n238 = Build Array (concatenate)(w187, w188) -> (w186:dbl[])
                                n239 = local write "VidStarted?"(TRUE ("VidStarted?")) -> ()
                                n240 = local write "loopTimes"(w190) -> ()
                              }
                            }
                          }
                        }
                      }
                      event User Event {
                        n241 = event-data() -> ("Event Data"=w198:bool)  [unwired: 1 in]
                        n242 = case shown="True" w198 {
                          tunnel: w197 -> [w201 w233]
                          tunnel: [w200 w233] -> w196
                          frame False {
                            n243 = flat-sequence {
                              tunnel: w201 -> [w202]
                              tunnel: [w227] -> w200
                              frame #0 {
                                n244 = local read "Avi Refnum"() -> (w226:T1)
                                n245 = local read "selected path"() -> (w219:path)
                                n246 = local write "Capture Video?"(FALSE ("Capture Video? 2")) -> ()
                                n247 = local write "VidStarted?"(FALSE ("VidStarted?")) -> ()
                                n248 = Path To String(path=w219) -> (string=w215:string)
                                n249 = call "IMAQ AVI Close"("Avi Refnum"=w226) -> ()  [unwired: 10 in, 1 out]
                                n250 = String Length(string=w215) -> (length=w214:i32)
                                n251 = Subtract(x=w214, y=4) -> (x-y=w212:i32)
                                n252 = local read "loopTimes"() -> (w225:dbl[])
                                n253 = String Subset(string=w215, offset (0)=0, length (rest)=w212) -> (substring=w203:string)
                                n254 = Concatenate Strings(w203, ".txt" ("string")) -> (w218:string)
                                n255 = Array To Spreadsheet String(delimiter (Tab)="\n", array=w202, 3:"%f" ("format string")) -> (spreadsheet string=w204:string)
                                n256 = Array To Spreadsheet String(delimiter (Tab)="\n", array=w225, 3:"%f" ("format string")) -> (spreadsheet string=w222:string)
                                n257 = Concatenate Strings(w203, "_pressure" ("string"), ".txt" ("string")) -> (w206:string)
                                n258 = String To Path(string=w206) -> (path=w205:path)
                                n259 = String To Path(string=w218) -> (path=w217:path)
                                n260 = Write to Text File(file (use dialog)=w217, text=w222) -> ()  [unwired: 2 in, 3 out]
                                n261 = Write to Text File(file (use dialog)=w205, text=w204) -> ()  [unwired: 2 in, 3 out]
                              }
                              frame #1 {
                                n262 = Initialize Array(0.0 ("element"), 1 ("dimension size")) -> (w227:dbl[])
                                n263 = Initialize Array(0.0 ("element"), 1 ("dimension size")) -> (w230:dbl[])
                                n264 = local write "loopTimes"(w230) -> ()
                              }
                            }
                          }
                          frame True {
                            n265 = flat-sequence {
                              frame #0 {
                                n266 = local read "FPS"() -> (w236:dbl)
                                n267 = call "File Dialog"() -> ("selected path"=w237:path)  [unwired: 12 in, 3 out]
                                "selected path" <- w237
                                n268 = Round To Nearest(number=w236) -> (nearest integer value=w235:dbl)
                                n269 = call "IMAQ AVI Create"("Frames Per Second"=w235, "AVI Path"=w237) -> ("Avi Refnum"=→"Avi Refnum":T1)  [unwired: 8 in, 1 out]
                              }
                              frame #1 {
                                n270 = local write "Capture Video?"(TRUE ("Capture Video? 2")) -> ()
                              }
                            }
                          }
                        }
                        n271 = Tick Count (ms) "FinalTick Count (ms)"() -> (millisecond timer value=w195:u32)
                      }
                      event "Accept ROI": Mouse Down; User Event {
                        n272 = event-data() -> ()  [unwired: 1 in, 2 out]
                        n273 = stacked-sequence {
                          tunnel: w239 -> [w252 _]
                          tunnel: w239 -> [_ w289]
                          frame #0 {
                            w273 = 32770 items=["IS_SET_IMAGE_AOI"=32770, "IS_GET_IMAGE_AOI"=32771] ("Mode")
                            # "Make sure x dim of ROI is div by 16\nand y dim is div by 2"
                            n274 = property on="ROI" class="ImageControl"() -> ("ROI"=w287:T7)  [unwired: 2 in, 2 out]
                            n275 = local read "ROI"() -> (w288:T2)
                            n276 = call "IMAQ ROIProfile"("ROI Descriptor"=w287, "Image"=w288) -> ("Global Rectangle"=w286:T8)  [unwired: 2 in, 4 out]
                            n277 = Unbundle By Name(w286) -> ("x1Left"=w272:i32, "y1Top"=w270:i32, "x2Right"=w271:i32, "y2Bottom"=w269:i32)
                            n278 = Subtract(x=w272, y=w271) -> (x-y=w285:i32)
                            n279 = Subtract(x=w270, y=w269) -> (x-y=w279:i32)
                            n280 = Absolute Value(x=w285) -> (abs(x)=w284:i32)
                            n281 = Absolute Value(x=w279) -> (abs(x)=w278:i32)
                            n282 = Max & Min(x=w270, y=w269) -> (min(x,y)=w258:i32)  [unwired: 1 out]
                            n283 = Max & Min(x=w272, y=w271) -> (min(x,y)=w257:i32)  [unwired: 1 out]
                            n284 = Divide(x=w284, y=16) -> (x/y=w282:dbl)
                            n285 = Divide(x=w278, y=2) -> (x/y=w276:dbl)
                            n286 = Round Toward -Infinity(1:w282) -> (0:w281:dbl)
                            n287 = Round Toward -Infinity(1:w276) -> (0:w275:dbl)
                            n288 = Multiply(x=w281, y=16.0) -> (x*y=w253:dbl)
                            "ROIXDim" <- w253
                            n289 = Multiply(x=w275, y=2.0) -> (x*y=w254:dbl)
                            "ROIYDim" <- w254
                            n290 = Absolute Value(x=w257) -> (abs(x)=w263:i32)
                            n291 = Absolute Value(x=w258) -> (abs(x)=w268:i32)
                            n292 = Divide(x=w263, y=16) -> (x/y=w261:dbl)
                            n293 = Divide(x=w268, y=2) -> (x/y=w266:dbl)
                            n294 = Round Toward -Infinity(1:w261) -> (0:w260:dbl)
                            n295 = Round Toward -Infinity(1:w266) -> (0:w265:dbl)
                            n296 = Multiply(x=w260, y=16.0) -> (x*y=w255:dbl)
                            n297 = Multiply(x=w265, y=2.0) -> (x*y=w256:dbl)
                            n298 = call "SetAOI.vi"("Camera Handle In"=w252, "Width In"=w253, "XPos In"=w255, "YPos In"=w256, "Mode"=w273, "Height In"=w254) -> ()  [unwired: 4 in, 6 out]
                          }
                          frame #1 {
                            n299 = call "GetImageSize.vi"("Camera Handle In"=w289) -> ("Height"=w295:i32, "Width"=w296:i32, "Camera Handle Out"=w293:u32)  [unwired: 8 in]
                            n300 = Bundle("Height"=w295, "Width"=w296) -> (w297:cluster{"Height":i32, "Width":i32})  [unwired: 1 in]
                            n301 = local read "Bits/Pixel"() -> (w290:i32)
                            n302 = local write "frameSize"(w297) -> ()
                            n303 = call "SetAllocatedImageMem.vi"("BitsPixel"=w290, "Height"=w295, "Width"=w296, "Camera Handle In"=w293) -> ("Image Memory Out"=w294:u8[], "Memory ID Out"=w291:i32, "Camera Handle Out"=w292:u32)  [unwired: 3 in, 2 out]
                            n304 = call "SetImageMem.vi"("Image Memory In"=w294, "Memory ID In"=w291, "Camera Handle In"=w292) -> ()  [unwired: 5 in, 4 out]
                          }
                        }
                        n305 = flat-sequence {
                          tunnel: [w244] -> w242
                          tunnel: w239 -> [w243]
                          tunnel: w242 -> [w249]
                          frame #0 {
                            n306 = call "GetActImgMem.vi"("Camera Handle In"=w243) -> ("Image Memory Out"=w244:u8[])  [unwired: 7 in, 3 out]
                          }
                          frame #1 {
                            # "Display Image"
                            n307 = local read "frameSize"() -> (w245:cluster{"Height":i32, "Width":i32})
                            n308 = Unbundle(w245) -> ("Height"=w247:i32, "Width"=w246:i32)
                            n309 = local read "ROI"() -> (w251:T2)
                            n310 = Reshape Array(w249, w247, w246) -> (w248:u8[][])
                            n311 = call "IMAQ ArrayToImage"("Image Pixels (U8)"=w248, "Image"=w251) -> ("Image Out"=w250:T2)  [unwired: 8 in, 1 out]
                            n312 = local write "ROI"(w250) -> ()
                          }
                        }
                        n313 = Tick Count (ms) "FinalTick Count (ms)"() -> (millisecond timer value=w240:u32)
                      }
                      event "Clear ROI": Mouse Down; User Event {
                        n314 = event-data() -> ()  [unwired: 1 in, 2 out]
                        n315 = stacked-sequence {
                          tunnel: w299 -> [w313 w321]
                          tunnel: [w312 _] -> w298
                          frame #0 {
                            w320 = 32770 items=["IS_SET_IMAGE_AOI"=32770, "IS_GET_IMAGE_AOI"=32771] ("Mode")
                            n316 = property on="ROI" class="ImageControl" props=["Image Area Size", "Image Area Height", "Image Area Width"]("Image Area Height"=u32 512 ("Image Area:Size:Height"), "Image Area Width"=u32 640 ("Image Area:Size:Width")) -> ()  [unwired: 2 in, 3 out]
                            n317 = call "SetAOI.vi"("Camera Handle In"=w313, "Width In"=1280, "XPos In"=0, "YPos In"=0, "Mode"=w320, "Height In"=1024) -> ("Camera Handle Out"=w312:u32)  [unwired: 4 in, 5 out]
                          }
                          frame #1 {
                            n318 = call "GetImageSize.vi"("Camera Handle In"=w321) -> ("Height"=w327:i32, "Width"=w328:i32, "Camera Handle Out"=w326:u32)  [unwired: 8 in]
                            n319 = local read "Bits/Pixel"() -> (w322:i32)
                            n320 = call "SetAllocatedImageMem.vi"("BitsPixel"=w322, "Height"=w327, "Width"=w328, "Camera Handle In"=w326) -> ("Image Memory Out"=w323:u8[], "Memory ID Out"=w324:i32, "Camera Handle Out"=w325:u32)  [unwired: 3 in, 2 out]
                            n321 = Bundle("Height"=w327, "Width"=w328) -> (w329:cluster{"Height":i32, "Width":i32})  [unwired: 1 in]
                            n322 = call "SetImageMem.vi"("Image Memory In"=w323, "Memory ID In"=w324, "Camera Handle In"=w325) -> ()  [unwired: 5 in, 4 out]
                            n323 = local write "frameSize"(w329) -> ()
                          }
                        }
                        n324 = flat-sequence {
                          tunnel: [w304] -> w302
                          tunnel: w298 -> [w303]
                          tunnel: w302 -> [w307]
                          frame #0 {
                            n325 = call "GetActImgMem.vi"("Camera Handle In"=w303) -> ("Image Memory Out"=w304:u8[])  [unwired: 7 in, 3 out]
                          }
                          frame #1 {
                            # "Display Image"
                            n326 = local read "frameSize"() -> (w305:cluster{"Height":i32, "Width":i32})
                            n327 = Unbundle(w305) -> ("Height"=w311:i32, "Width"=w310:i32)
                            n328 = Reshape Array(w307, w311, w310) -> (w306:u8[][])
                            n329 = local read "ROI"() -> (w309:T2)
                            n330 = call "IMAQ ArrayToImage"("Image Pixels (U8)"=w306, "Image"=w309) -> ("Image Out"=w308:T2)  [unwired: 8 in, 1 out]
                            n331 = local write "ROI"(w308) -> ()
                          }
                        }
                        n332 = Tick Count (ms) "FinalTick Count (ms)"() -> (millisecond timer value=w300:u32)
                      }
                    }
                    n333 = local read "Frame rate"() -> (w96:dbl)
                    n334 = local read "stop"() -> (w89:bool)
                    n335 = Reciprocal(x=w96) -> (1/x=w97:dbl)
                    n336 = Multiply(x=w97, y=1000) -> (x*y=w99:dbl)
                    n337 = Or(x=w89, y="Stopp") -> (x .or. y?=w90:bool)
                    n338 = Wait Until Next ms Multiple(millisecond multiple=w99) -> ()  [unwired: 1 out]
                  }
                }
                frame Error {
                }
              }
            }
            frame #2 {
              # "Stop Capture"
              n339 = call "StopLiveVideo.vi"("Camera Handle In"=w334) -> ("error out"=w332:errorcluster, "Camera Handle Out"=w333:u32)  [unwired: 9 in]
              n340 = local read "Capture Video?"() -> (w331:bool)
              n341 = case shown="True" w331 {
                frame False {
                }
                frame True {
                  n342 = local read "Avi Refnum"() -> (w341:T1)
                  n343 = call "IMAQ AVI Close"("Avi Refnum"=w341) -> ()  [unwired: 10 in, 1 out]
                  n344 = local write "VidStarted?"(FALSE ("VidStarted?")) -> ()
                  n345 = local write "Capture Video?"(FALSE ("Capture Video?")) -> ()
                  n346 = local read "loopTimes"() -> (w336:dbl[])
                  n347 = Array To Spreadsheet String(delimiter (Tab)="\n", array=w336, 3:"%f" ("format string")) -> (spreadsheet string=w337:string)
                  n348 = Write to Text File(text=w337) -> ()  [unwired: 3 in, 3 out]
                }
              }
            }
          }
        }
      }
      "error out" <- w34
      n349 = Unregister For Events(event registration refnum=w32) -> ()  [unwired: 1 in, 1 out]
      n350 = call "ExitCamera.vi"("error in"=w34, "Camera Handle In"=w38) -> ()  [unwired: 9 in, 1 out]
    }
  }
  n351 = call <vilib>:"General Error Handler.vi"("error in (no error)"=w18) -> ()  [unwired: 1 in, 14 out]
  "PressureOffset" <- 0.0 ("PressureOffset")
  "VidStarted?" <- FALSE ("VidStarted?")
  "Capture Video? 2" <- FALSE ("Capture Video? 2")
